vi "main.vi"() -> ()   [LabVIEW 2013]
doc: "Use this template to build a producer/consumer design pattern with events to produce queue items. Use this design pattern instead of the User Interface Event Handler pattern for user interfaces when you want to execute code asynchronously in response to an event without slowing the user interface responsiveness."
uses:
  Microscope_Settings.ctl
  Laser.ctl
  Time_microseconds.ctl
  Phase_Shift.ctl
  Mirror_Voltage.ctl
  Z_Offset.ctl
  Gain.ctl
  Tuneable_Lens_Numeric_Control.ctl
  Piezo_micrometres.ctl
  waveforms.ctl
  Piezo_micrometres_slider_control.ctl
  Mirror_Gain_Slider_Control.ctl
  Tunable_Lens_Slider_Control.ctl
panel:
  in  "COM port":i32
  in  "Filter Wheel Position":i32
  in  "Mode":T1(ring)
  in  "Number of Repetitions":u16=1 min=1 step=1
  in  "Time Interval  Between Repeats (µS)":T2 step=2
  in  "StopMultiDScan":bool
  in  "StartMultiDScan":bool
  in  "Number of Z Slices":i16=1 min=1 step=1
  in  "Z Mirror Control":enum16{"manual", "automatic"}(ring)
  in  "Apply ex/det correction":enum16{"no", "yes"}(ring)
  out "Z Mirror Voltage":T3 min=-10.0 max=10.0
  out "Adjusted Scan Mirror Voltage":T3 min=-10.0 max=10.0
  in  "set@minZ":bool
  in  "set@maxZ":bool
  in  "@ min Z":T3 min=-10.0 max=10.0
  in  "@ max Z":T3 min=-10.0 max=10.0
  in  "PiezoEndMicrometres":T4 caption="End (µm)" min=0.0 max=100.0
  in  "PiezoStartMicrometres":T4 caption="Start (µm)" min=0.0 max=100.0
  in  "setPiezoEnd":bool
  in  "setPiezoStart":bool
  in  "Lens 2":T5 min=0.0 max=3.0 step=0.0001 scale=0.0..3.0
  in  "Lens 1":T5 min=0.0 max=3.0 step=0.0001 scale=0.0..3.0
  in  "saveMicroscopeSettings":bool
  in  "applyCurrentMicroscopeSettings":bool
  in  "deleteCurrentMicroscopeSettings":bool
  in  "loadMicroscopeSettings":bool
  in  "addMicroscopeSettings":bool
  in  "Z Mirror Gain":T6 min=-10.0 max=10.0 scale=-10.0..10.0
  in  "Mirror Offset":dbl(slide) min=-10.0 max=10.0 step=0.01 scale=-10.0..10.0
  in  "Laser":T7
  in  "Piezo Position (µm)":T8 min=0.0 max=100.0 scale=0.0..100.0
  in  "Mirror Voltage":dbl(slide) min=-10.0 max=10.0 step=0.01 scale=-10.0..10.0
  in  "setPosition2":bool
  in  "setPosition1":bool
  in  "Z offset 2":T9
  in  "Z offset 1":T9
  in  "Scan Mirror 2":T3 min=-10.0 max=10.0
  in  "Scan Mirror 1":T3 min=-10.0 max=10.0
  in  "setScanMirrorMin":bool
  in  "setScanMirrorMax":bool
  in  "MinScanMirror":T3 caption="Min" min=-10.0 max=10.0
  in  "MaxScanMirror":T3 caption="Max" min=-10.0 max=10.0
  in  "Offset":T3 min=-10.0 max=10.0
  in  "Amplitude":T3 min=-10.0 max=10.0
  in  "Phase Shift (µS)":i32(slide) scale=-5000.0..1000.0
  in  "Sweep Interval (µS)":T2 step=2
  in  "Sweep Time (µS)":T2 step=20
  in  "Microscope Settings":T10[](array[typedef]) {"Number Z Slices" min=1 step=1; "Piezo End (µm)" min=0.0 max=100.0; "Piezo Start (µm)" min=0.0 max=100.0; "Beam @ max Z" min=-10.0 max=10.0; "Beam @ min Z" min=-10.0 max=10.0; "Tuneable Lens 2" min=0.0 max=3.0 step=0.0001; "Tuneable Lens 1" min=0.0 max=3.0 step=0.0001; "Scan Mirror Position 2" min=-10.0 max=10.0; "Scan Mirror Position 1" min=-10.0 max=10.0; "Scan Mirror Amplitude" min=-10.0 max=10.0; "Scan Mirror Min" min=-10.0 max=10.0; "Scan Mirror Max" min=-10.0 max=10.0; "Sweep Interval (µS)" step=2; "Sweep Time (µS)" step=2}
  in  "Sample Rate (kHz)":i32
  in  "StopSinglePlaneScan":bool
  in  "StartSinglePlaneScan":bool
  in  "exit":bool
  # "Piezo Settings"
  # "Scan Mirror Settings"
  # "Z Mirror Local Settings"
  # "Single Plane Scan"
  # "Multidimensional Scan"
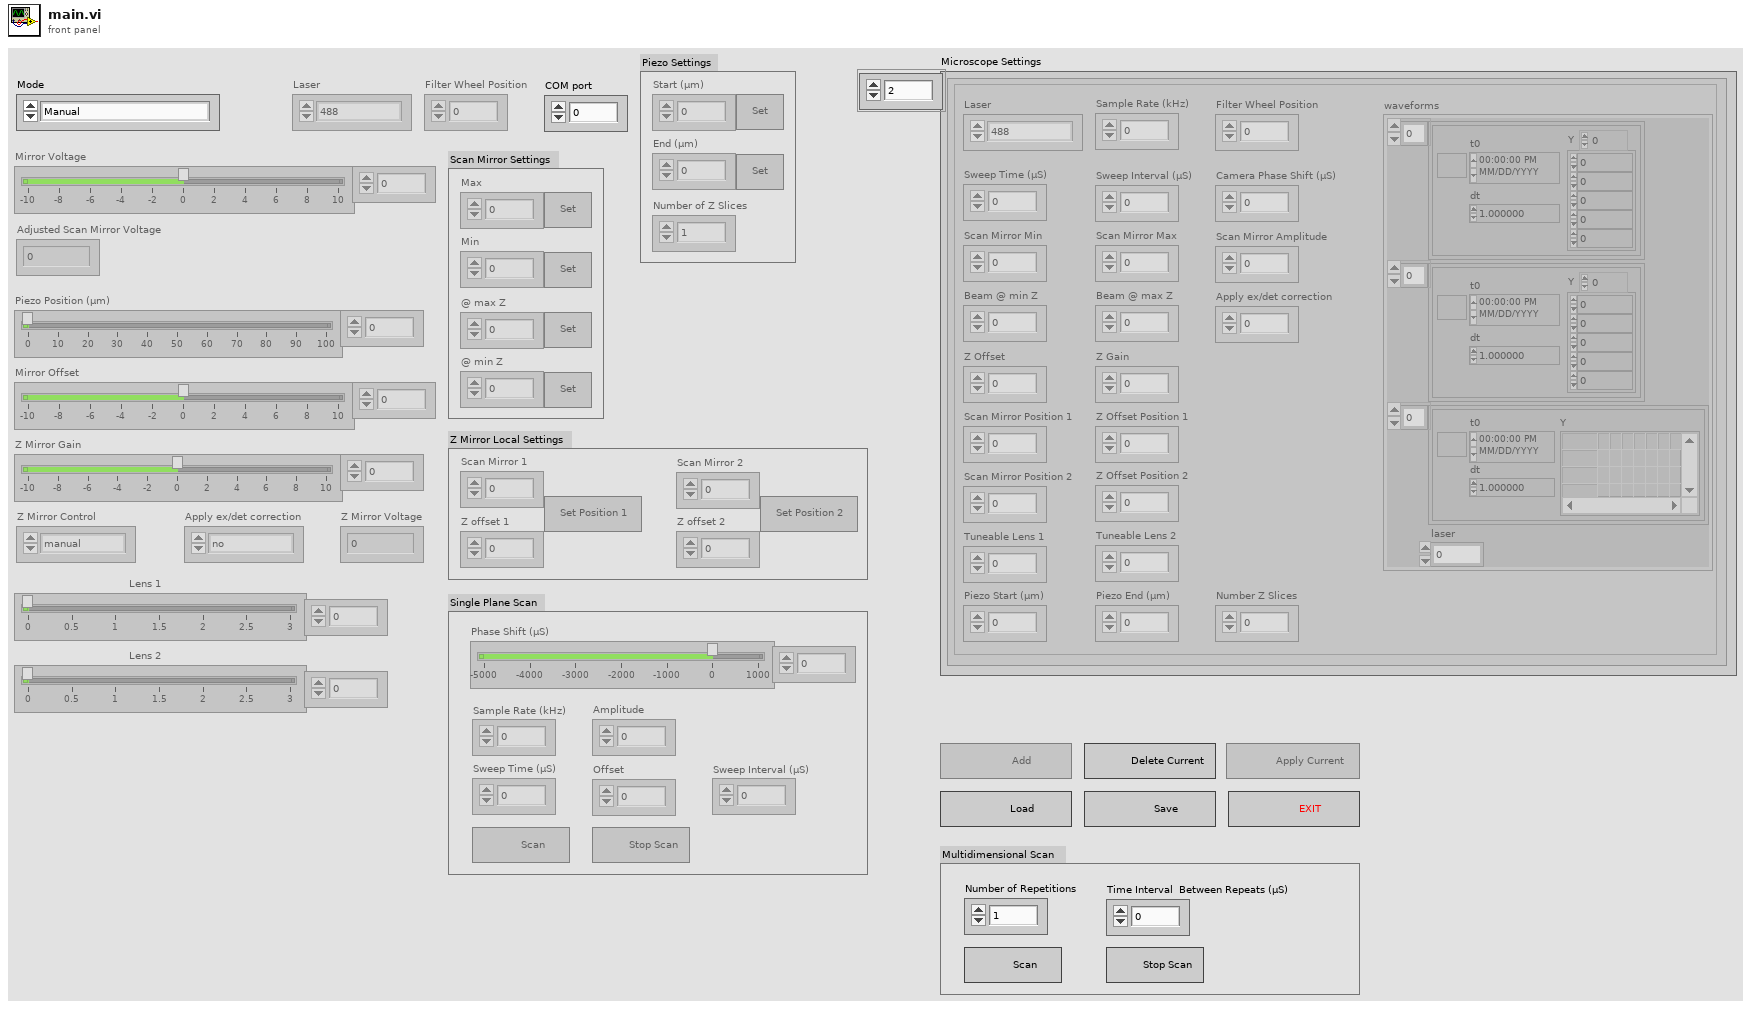
[diagram p1: front panel]
types:
  T1 = enum8{"Manual", "Single Plane Scan", "Multi-Dimensional Scan"}
  T2 = typedef "Time_microseconds.ctl" = u32
  T3 = typedef "Mirror_Voltage.ctl" = dbl
  T4 = typedef "Piezo_micrometres.ctl" = dbl
  T5 = typedef "Tunable_Lens_Slider_Control.ctl" = dbl
  T6 = typedef "Mirror_Gain_Slider_Control.ctl" = dbl
  T7 = typedef "Laser.ctl" = enum16{"488", "561"}
  T8 = typedef "Piezo_micrometres_slider_control.ctl" = dbl
  T9 = typedef "Z_Offset.ctl" = dbl
  T10 = typedef "Microscope_Settings.ctl" = cluster{"Laser":T7, "Sweep Time (µS)":T2, "Sweep Interval (µS)":T2, "Sample Rate (kHz)":dbl, "Camera Phase Shift (µS)":T11, "Scan Mirror Max":T3, "Scan Mirror Min":T3, "Scan Mirror Amplitude":T3, "Z Offset":T9, "Z Gain":T12, "Scan Mirror Position 1":T3, "Z Offset Position 1":T9, "Scan Mirror Position 2":T3, "Z Offset Position 2":T9, "Tuneable Lens 1":T13, "Tuneable Lens 2":T13, "Beam @ min Z":T3, "Beam @ max Z":T3, "Piezo Start (µm)":T4, "Piezo End (µm)":T4, "Number Z Slices":i16, "Filter Wheel Position":i32, "Apply ex/det correction":u16, "waveforms":T14}
  T11 = typedef "Phase_Shift.ctl" = i32
  T12 = typedef "Gain.ctl" = dbl
  T13 = typedef "Tuneable_Lens_Numeric_Control.ctl" = dbl
  T14 = typedef "waveforms.ctl" = cluster{waveform(dbl)[], waveform(dbl)[], digitalwaveform[], "laser":i32}
  T15 = enum8{"Enabled", "Disabled", "Disabled and Grayed Out"}
  T16 = enum16{"deny read/write", "deny write-only", "deny none"}
  T17 = enum16{"open", "replace", "create", "open or create", "replace or create", "replace or create with confirmation"}
  T18 = cluster{"Laser":T7, "Sweep Time (µS)":T2, "Sweep Interval (µS)":T2, "Sample Rate (kHz)":i32, "Phase Shift (µS)":i32, "MaxScanMirror":T3, "MinScanMirror":T3, "MaxScanMirror":T3, "Mirror Offset":dbl, "Z Mirror Gain":T6, "Scan Mirror 1":T3, "Z offset 1":T9, "Scan Mirror 2":T3, "Z offset 2":T9, "Lens 1":T5, "Lens 2":T5, "@ min Z":T3, "@ max Z":T3, "PiezoStartMicrometres":T4, "PiezoEndMicrometres":T4, "Number of Z Slices":i16, "Filter Wheel Position":i32, "Apply ex/det correction":enum16{"no", "yes"}}
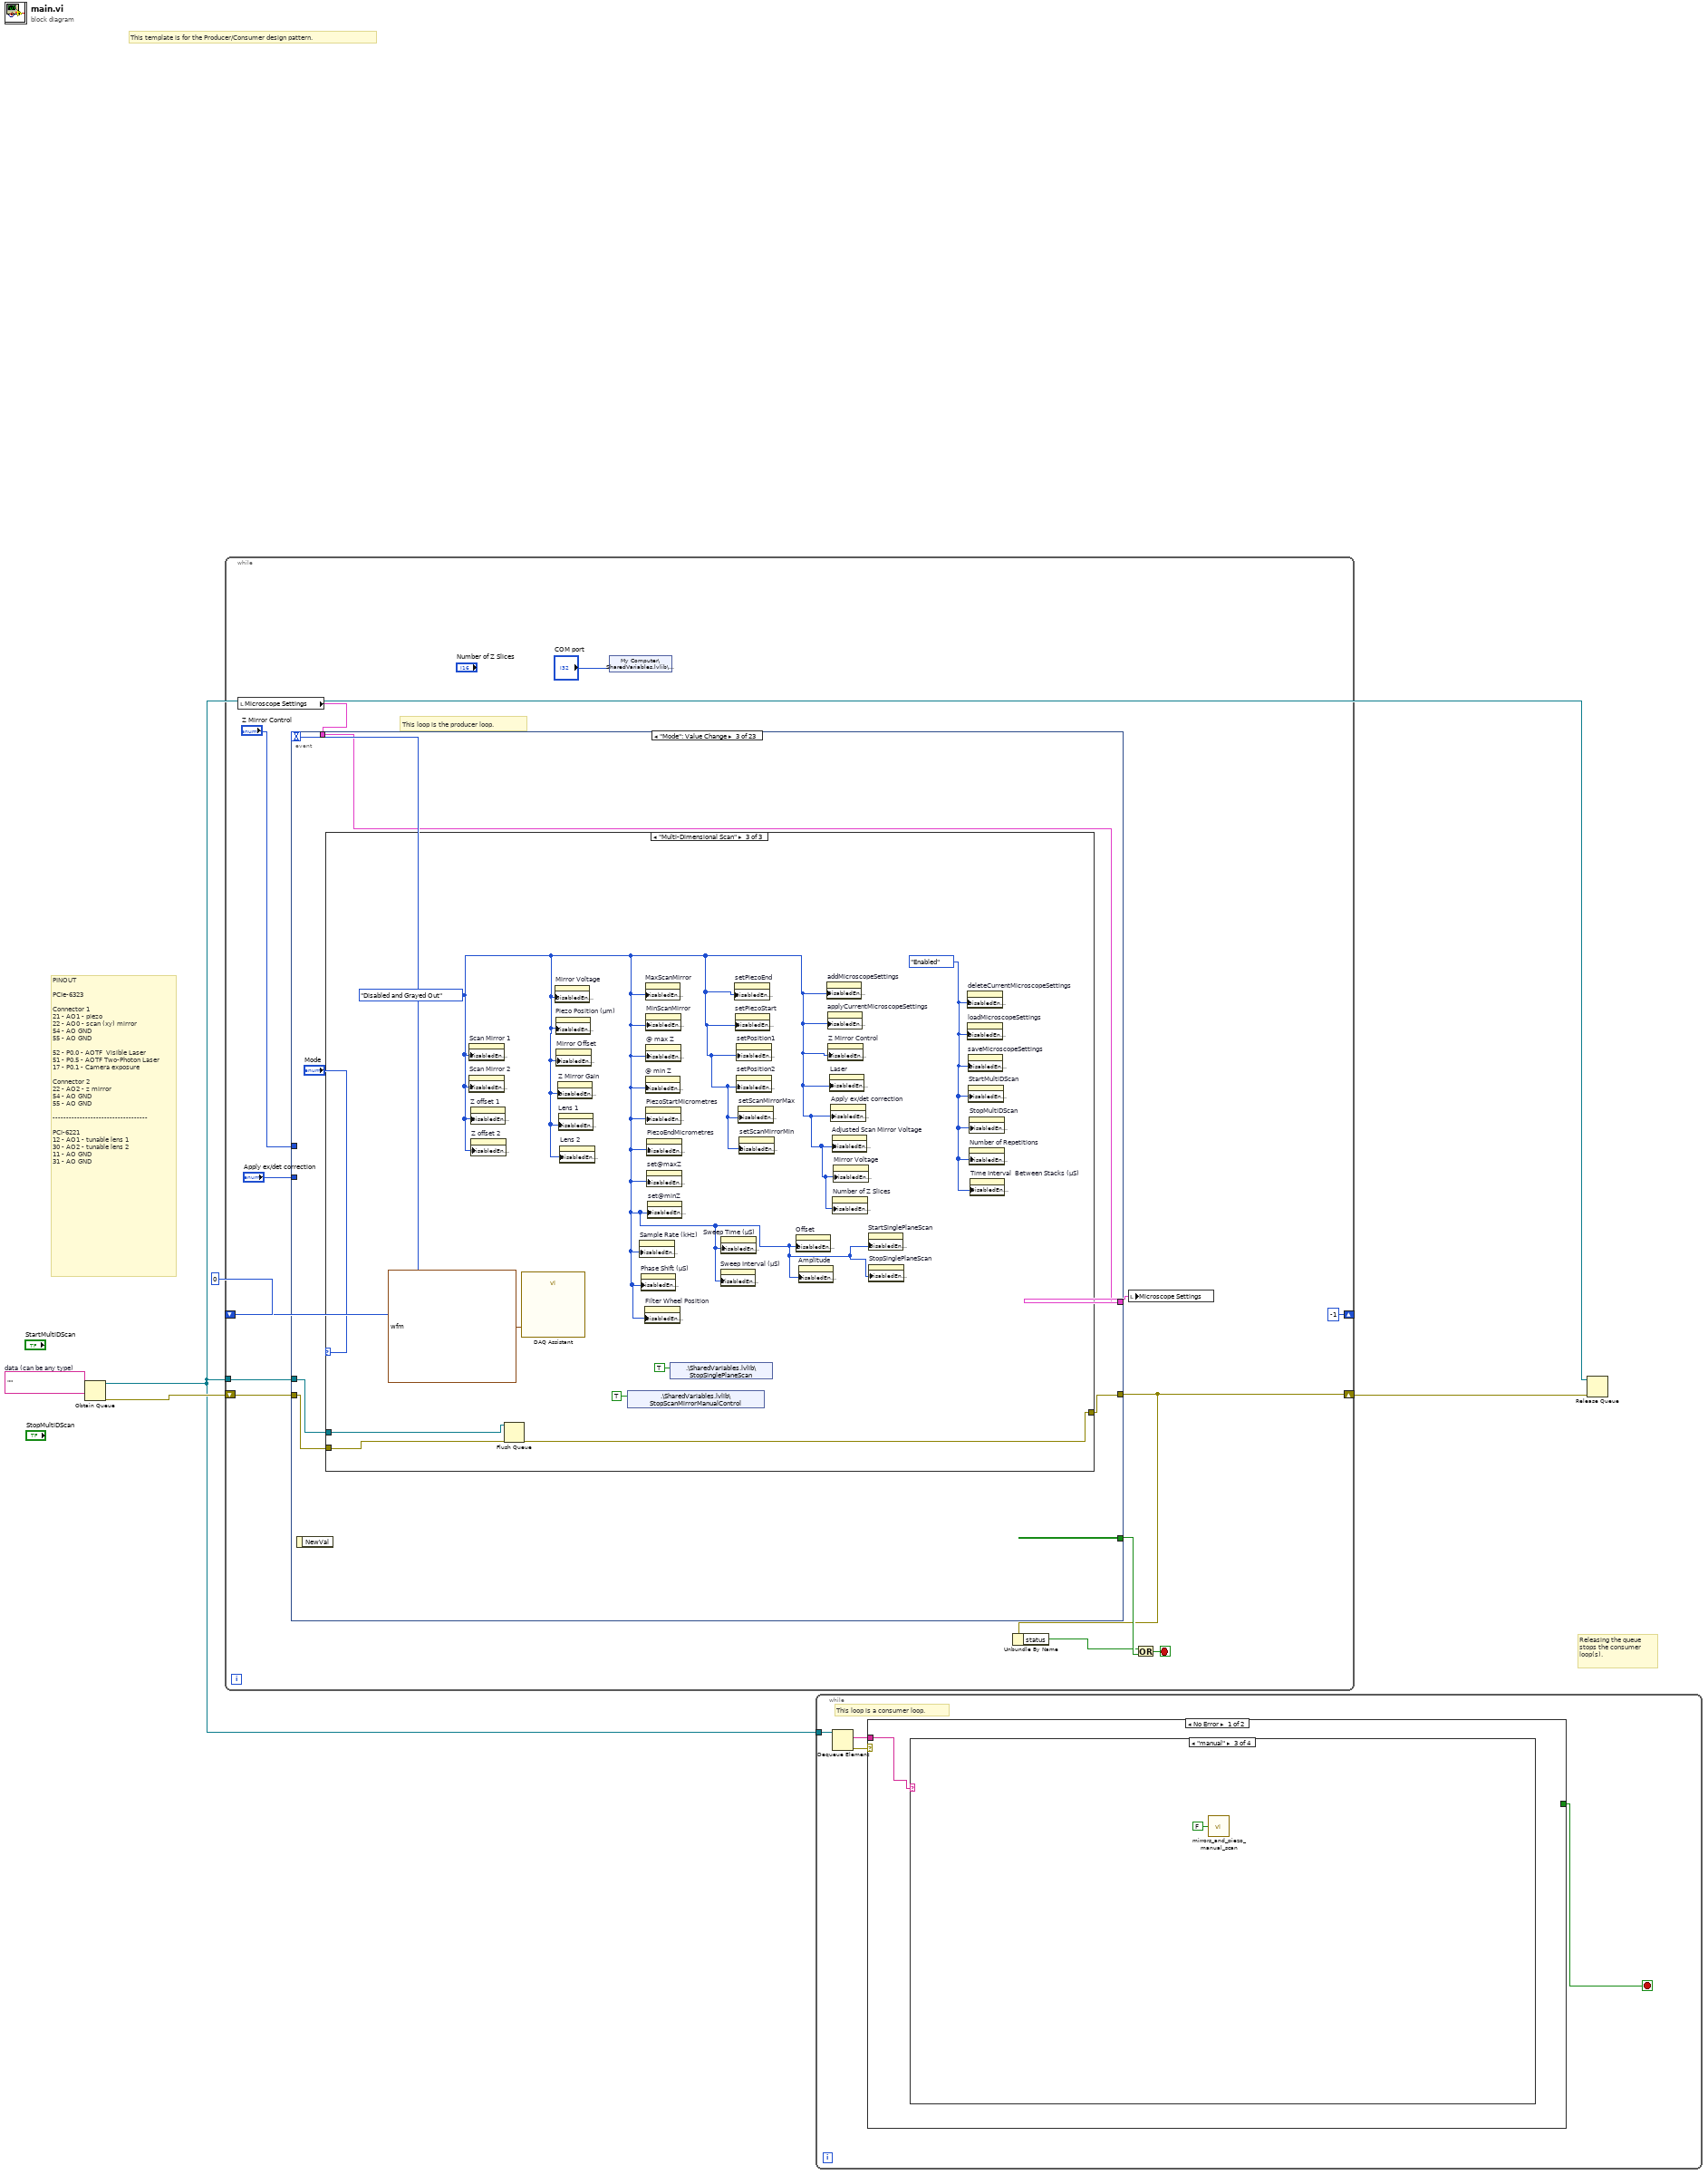
[diagram p0: block diagram]
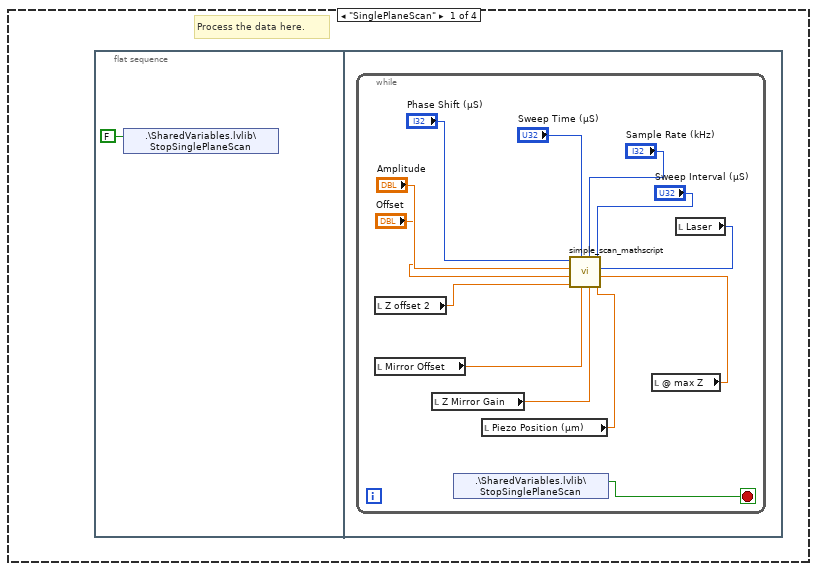
[diagram p2: hidden frame]
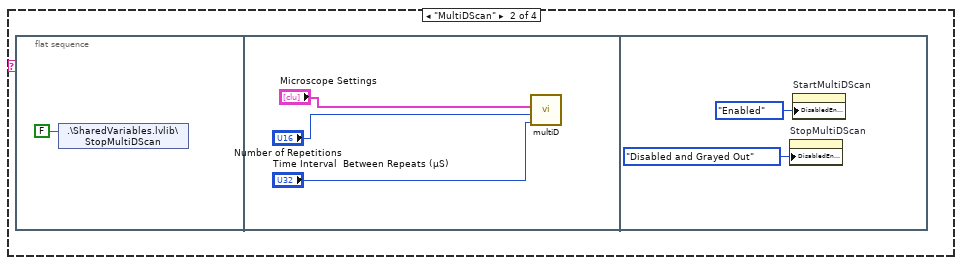
[diagram p3: hidden frame]
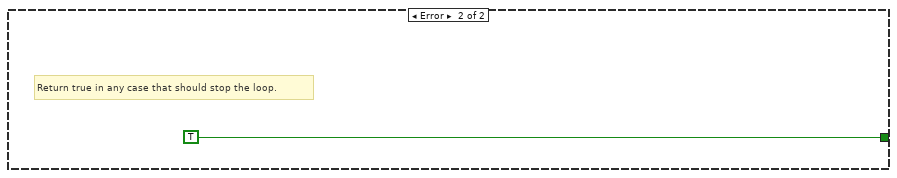
[diagram p5: hidden frame]
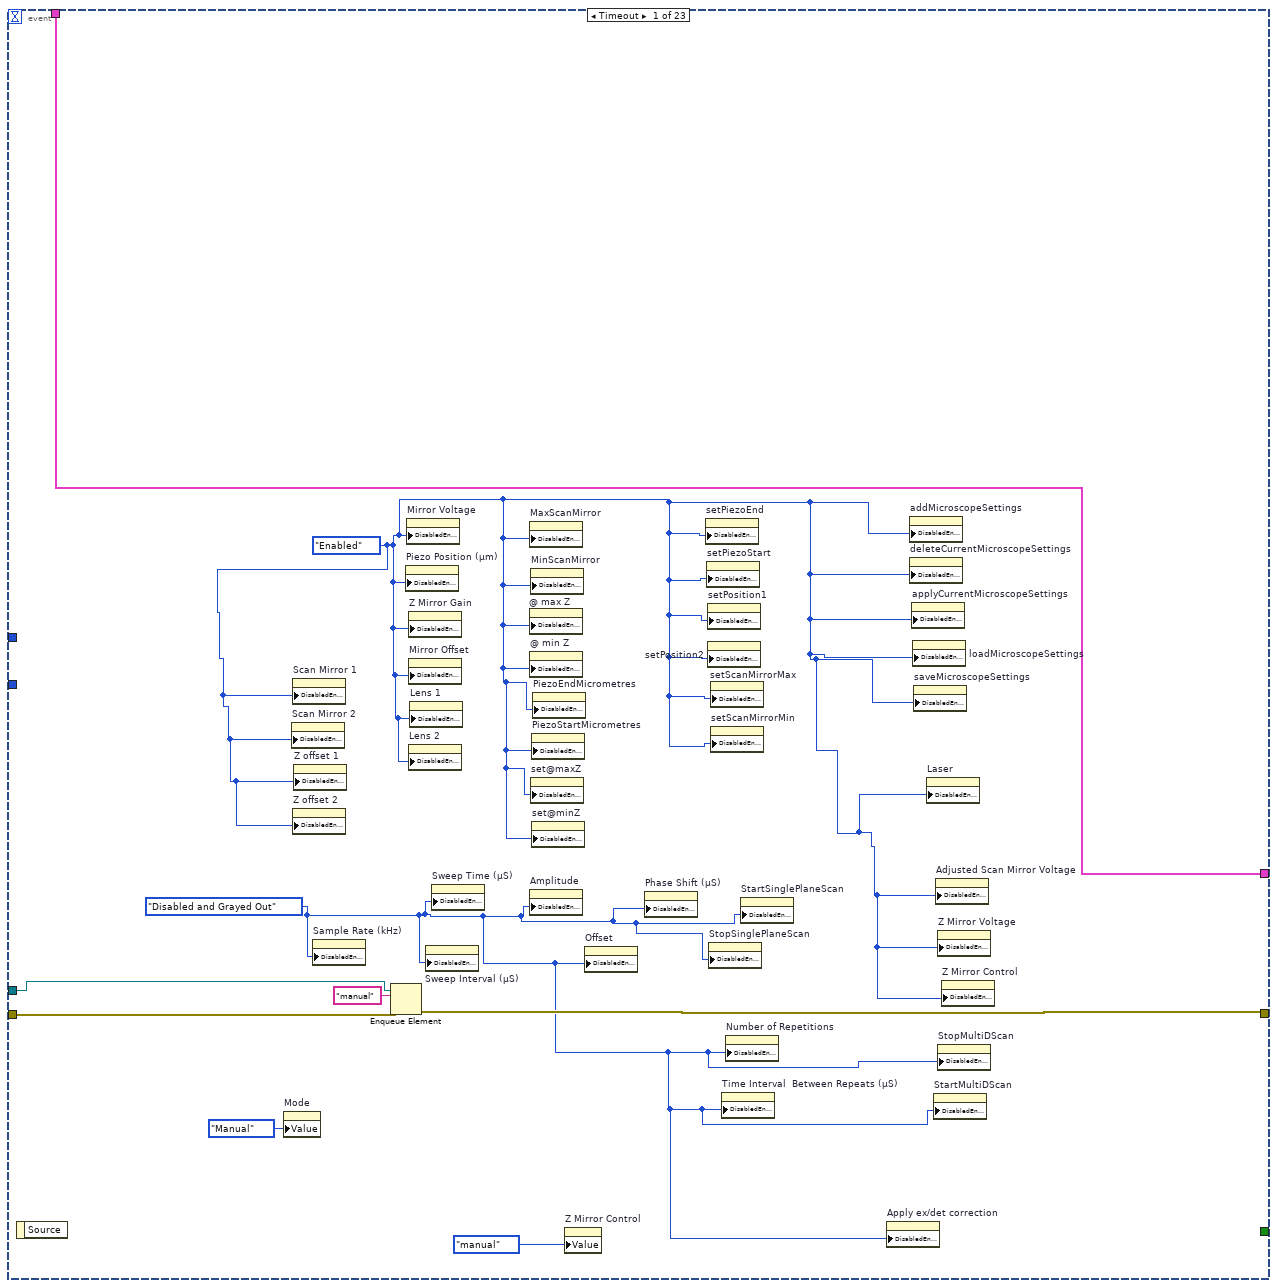
[diagram p6: hidden frame]
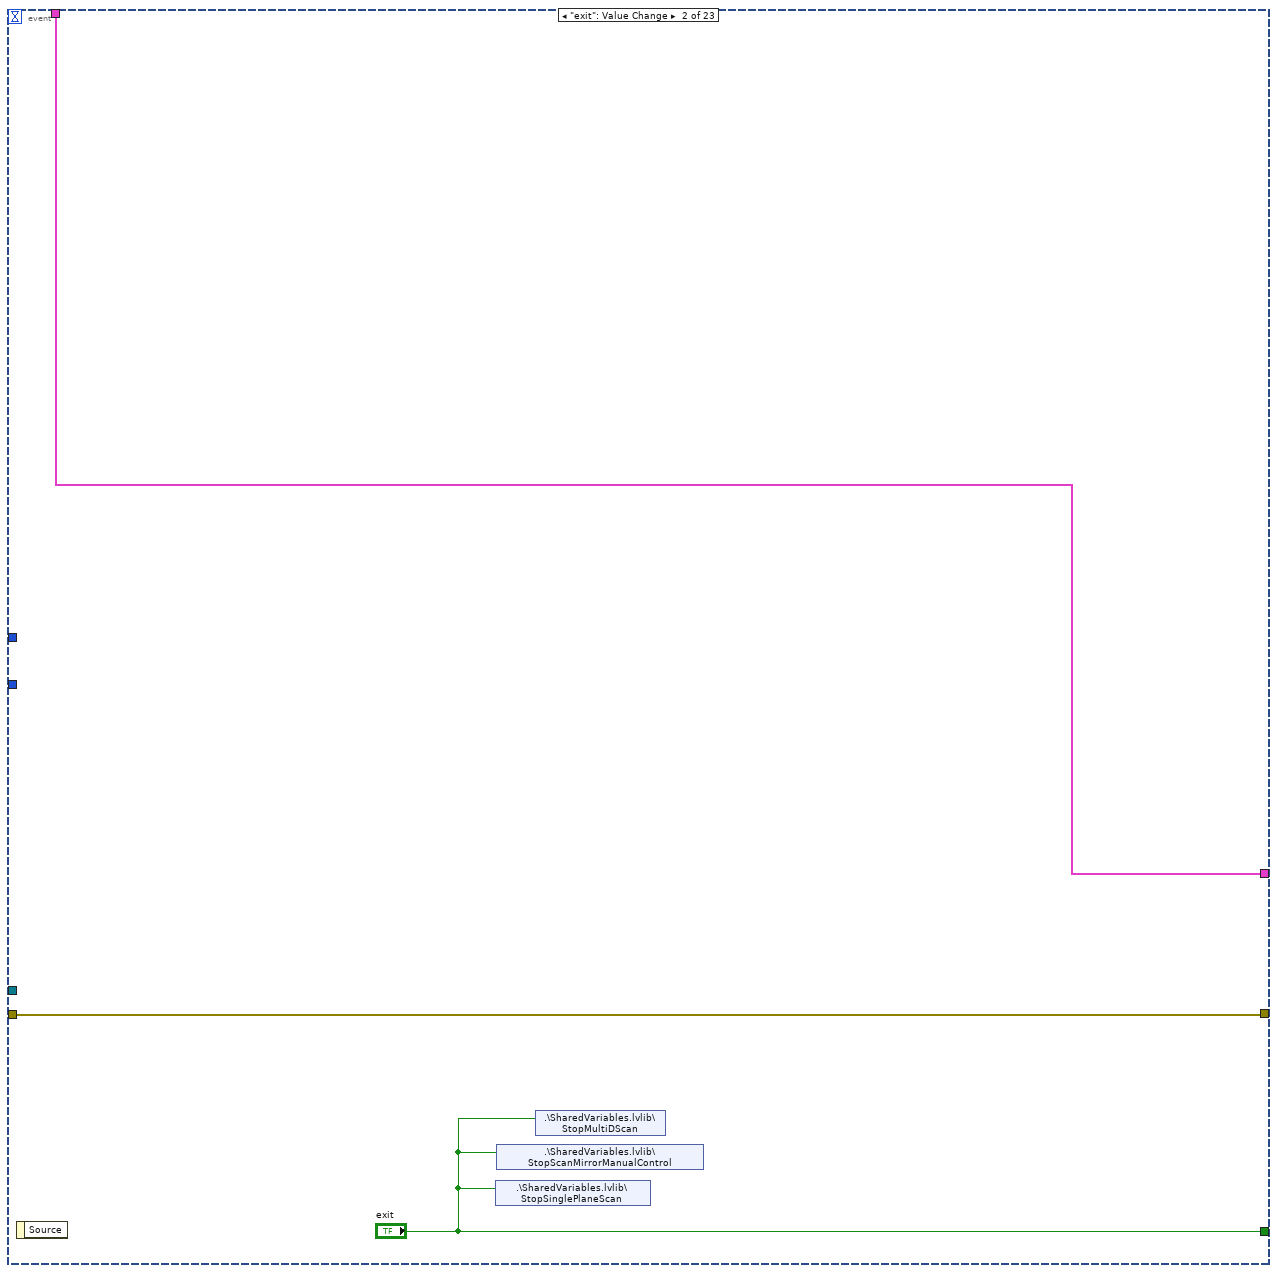
[diagram p7: hidden frame]
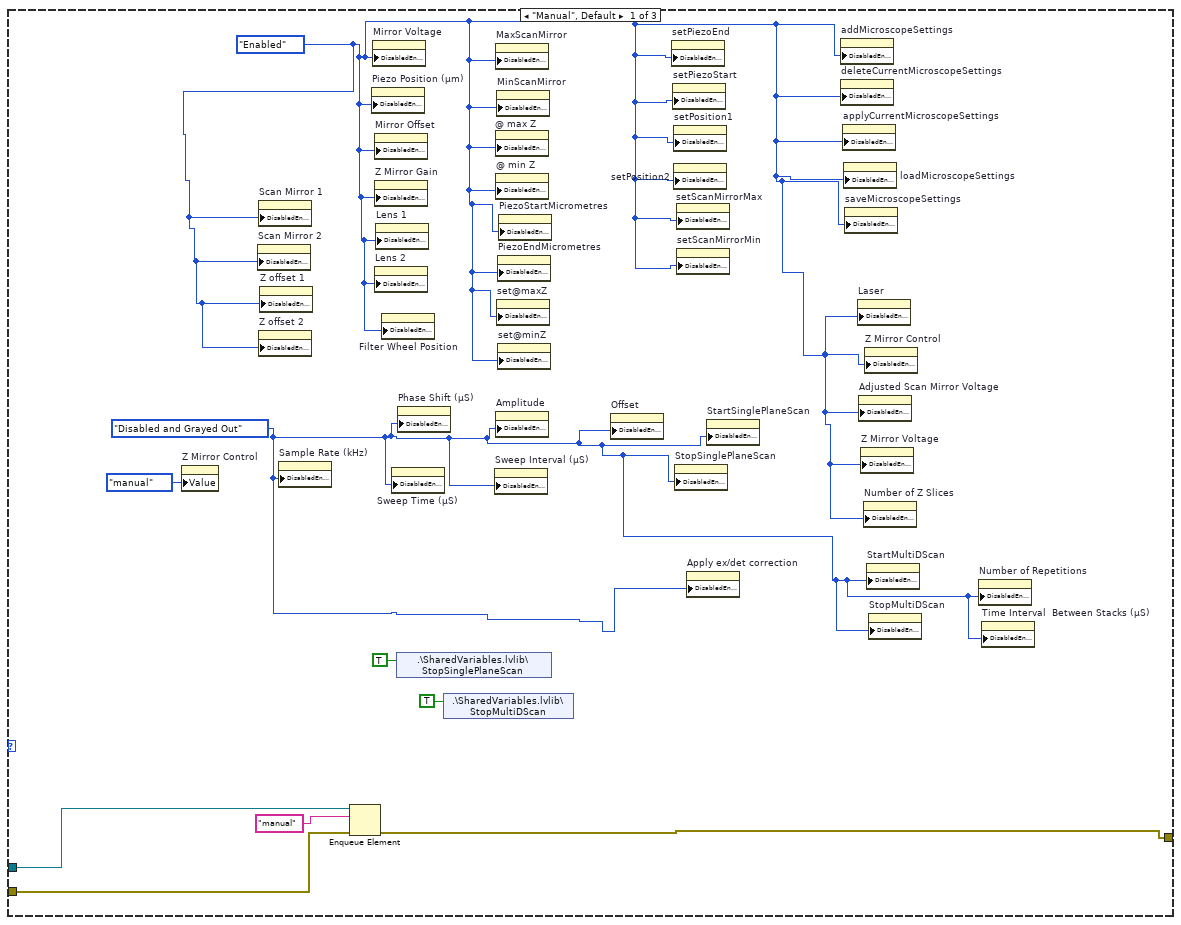
[diagram p8: hidden frame]
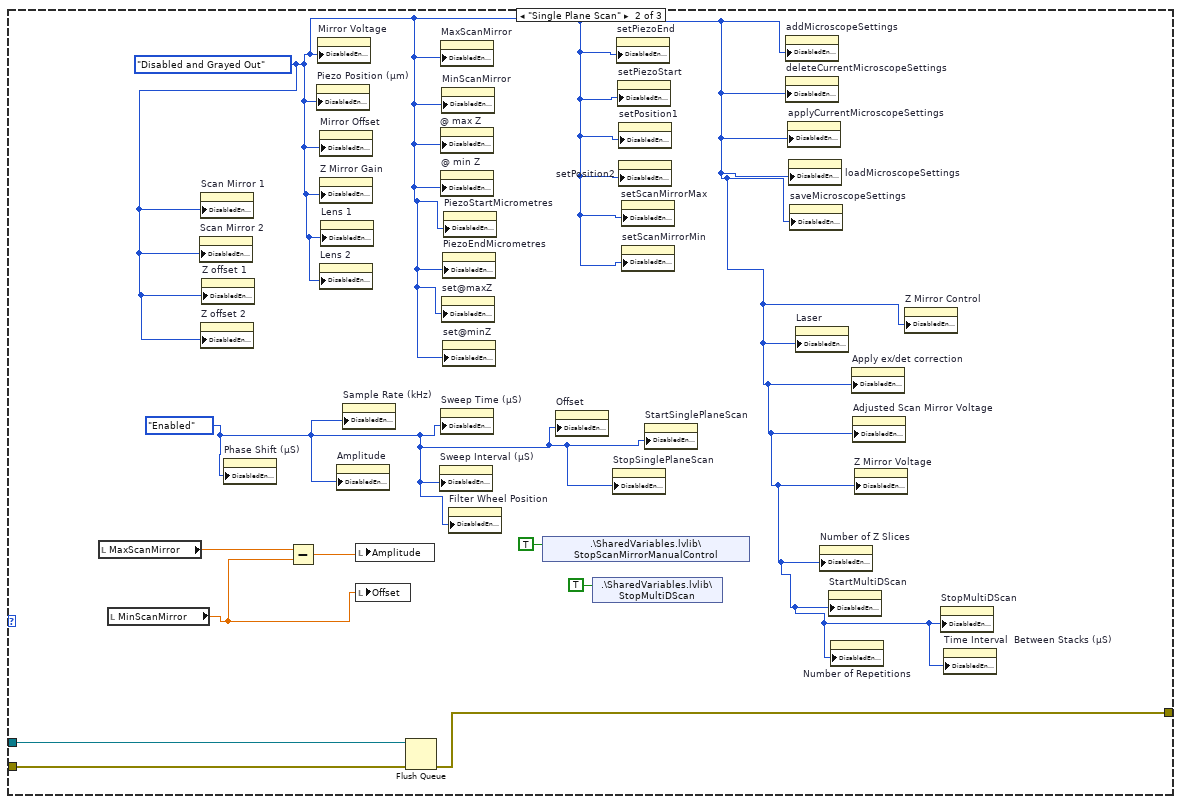
[diagram p9: hidden frame]
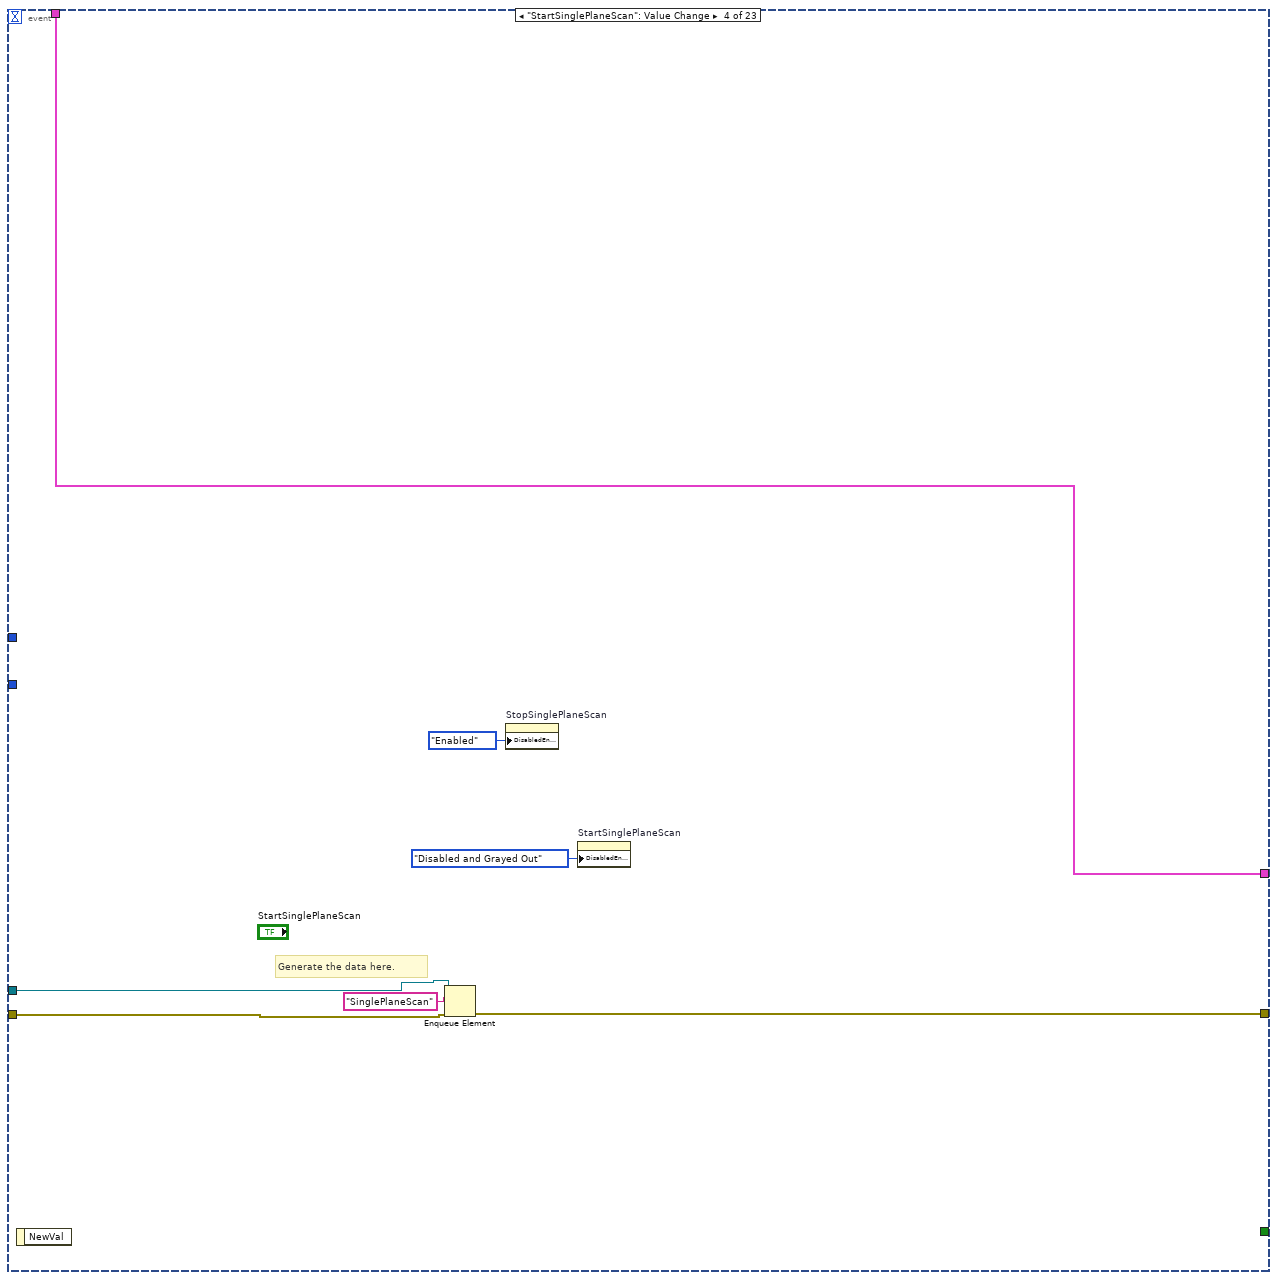
[diagram p10: hidden frame]
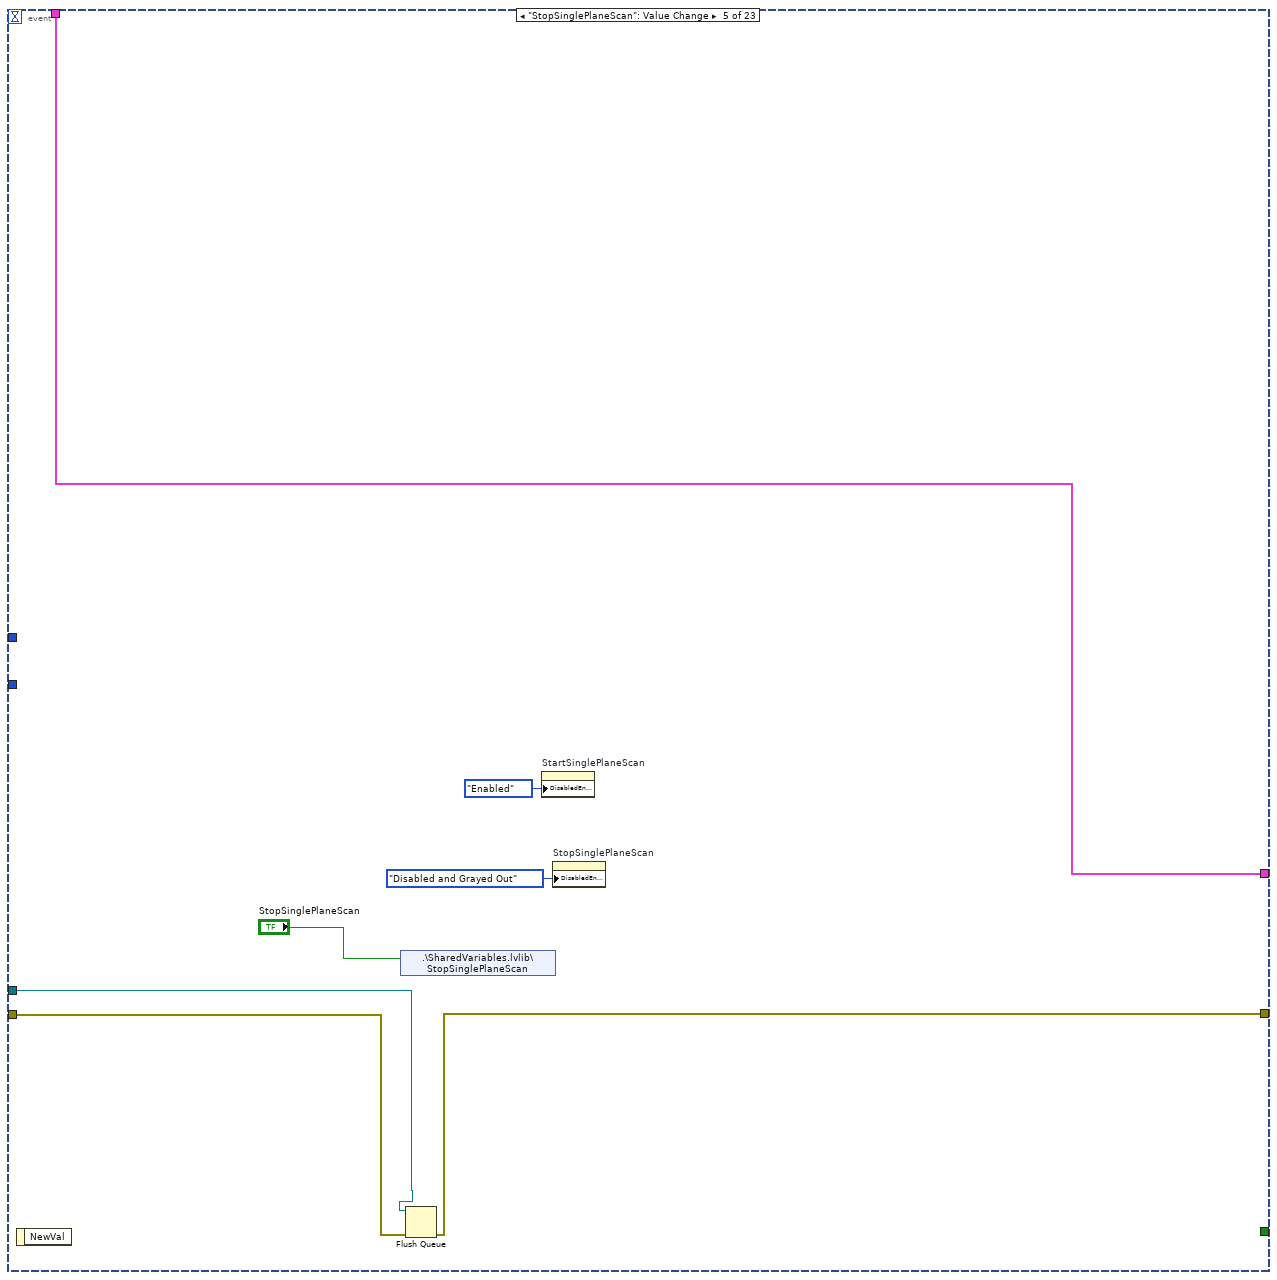
[diagram p11: hidden frame]
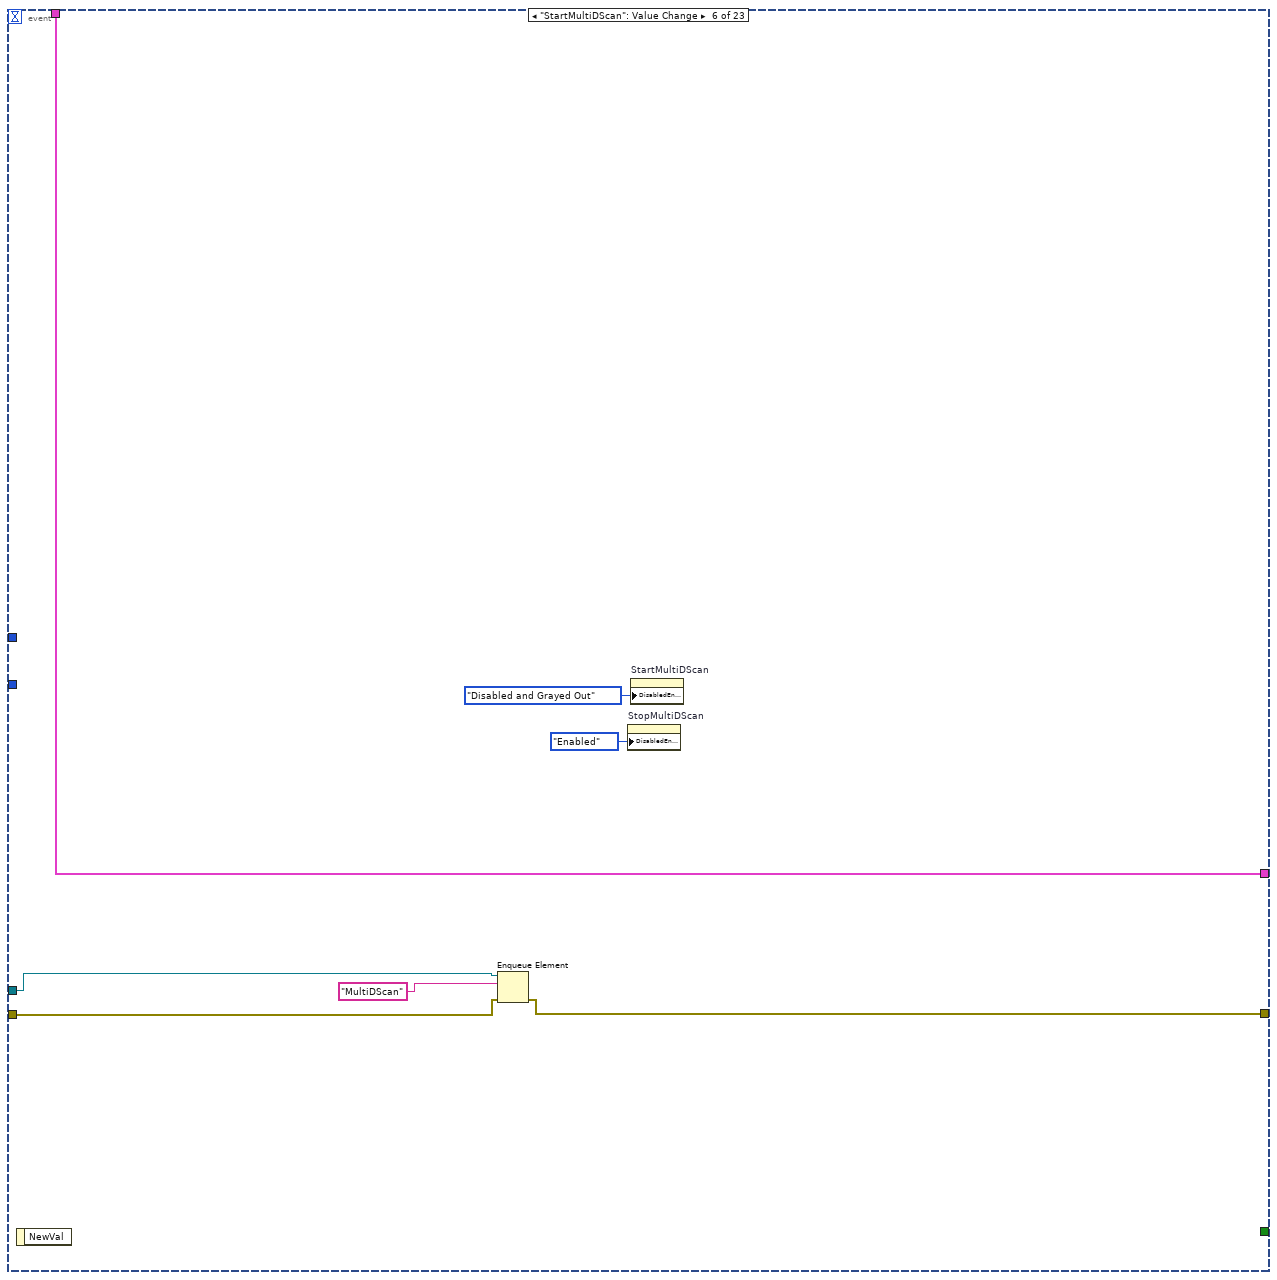
[diagram p12: hidden frame]
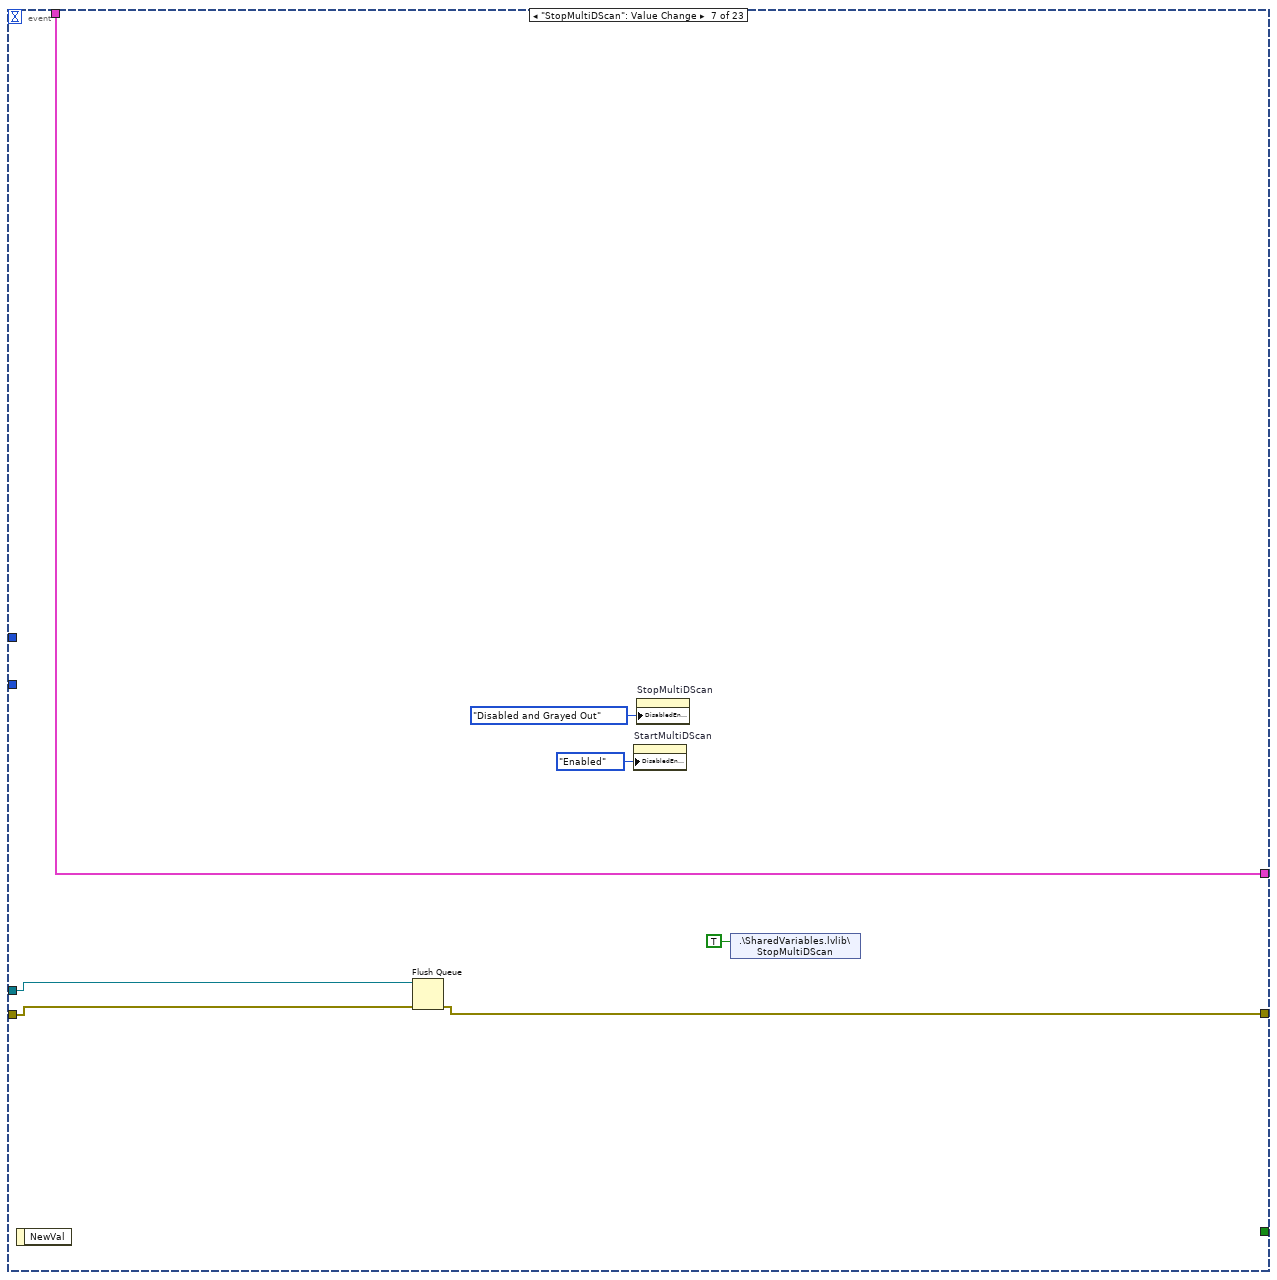
[diagram p13: hidden frame]
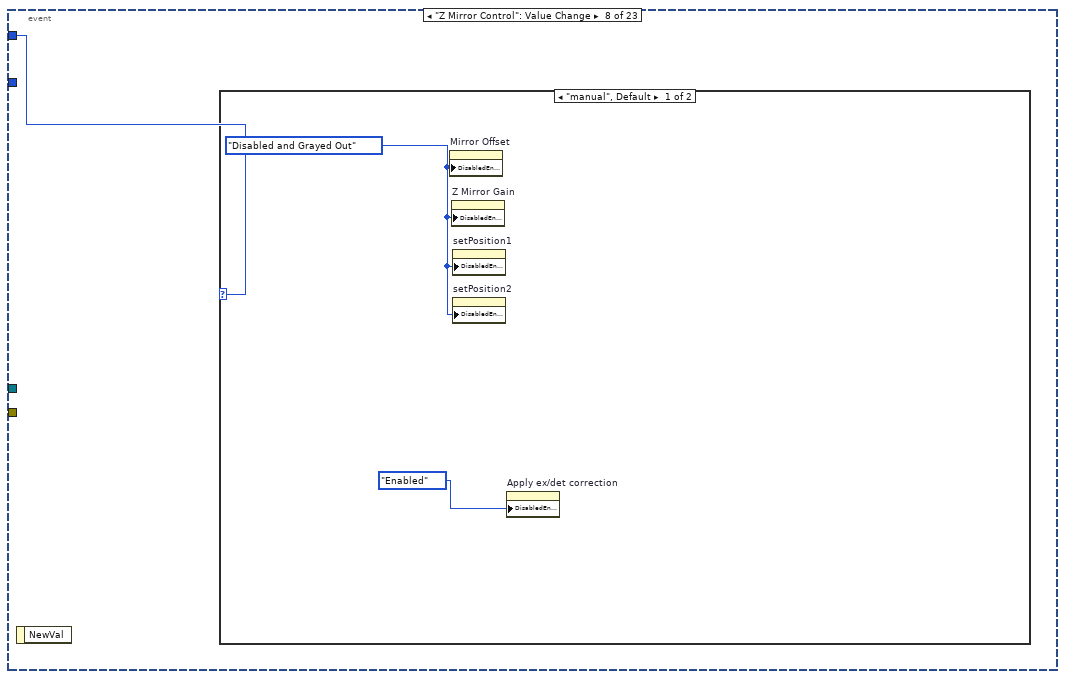
[diagram p14: hidden frame]
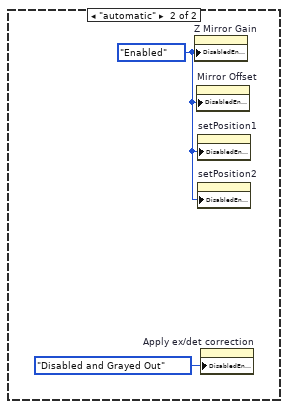
[diagram p15: hidden frame]
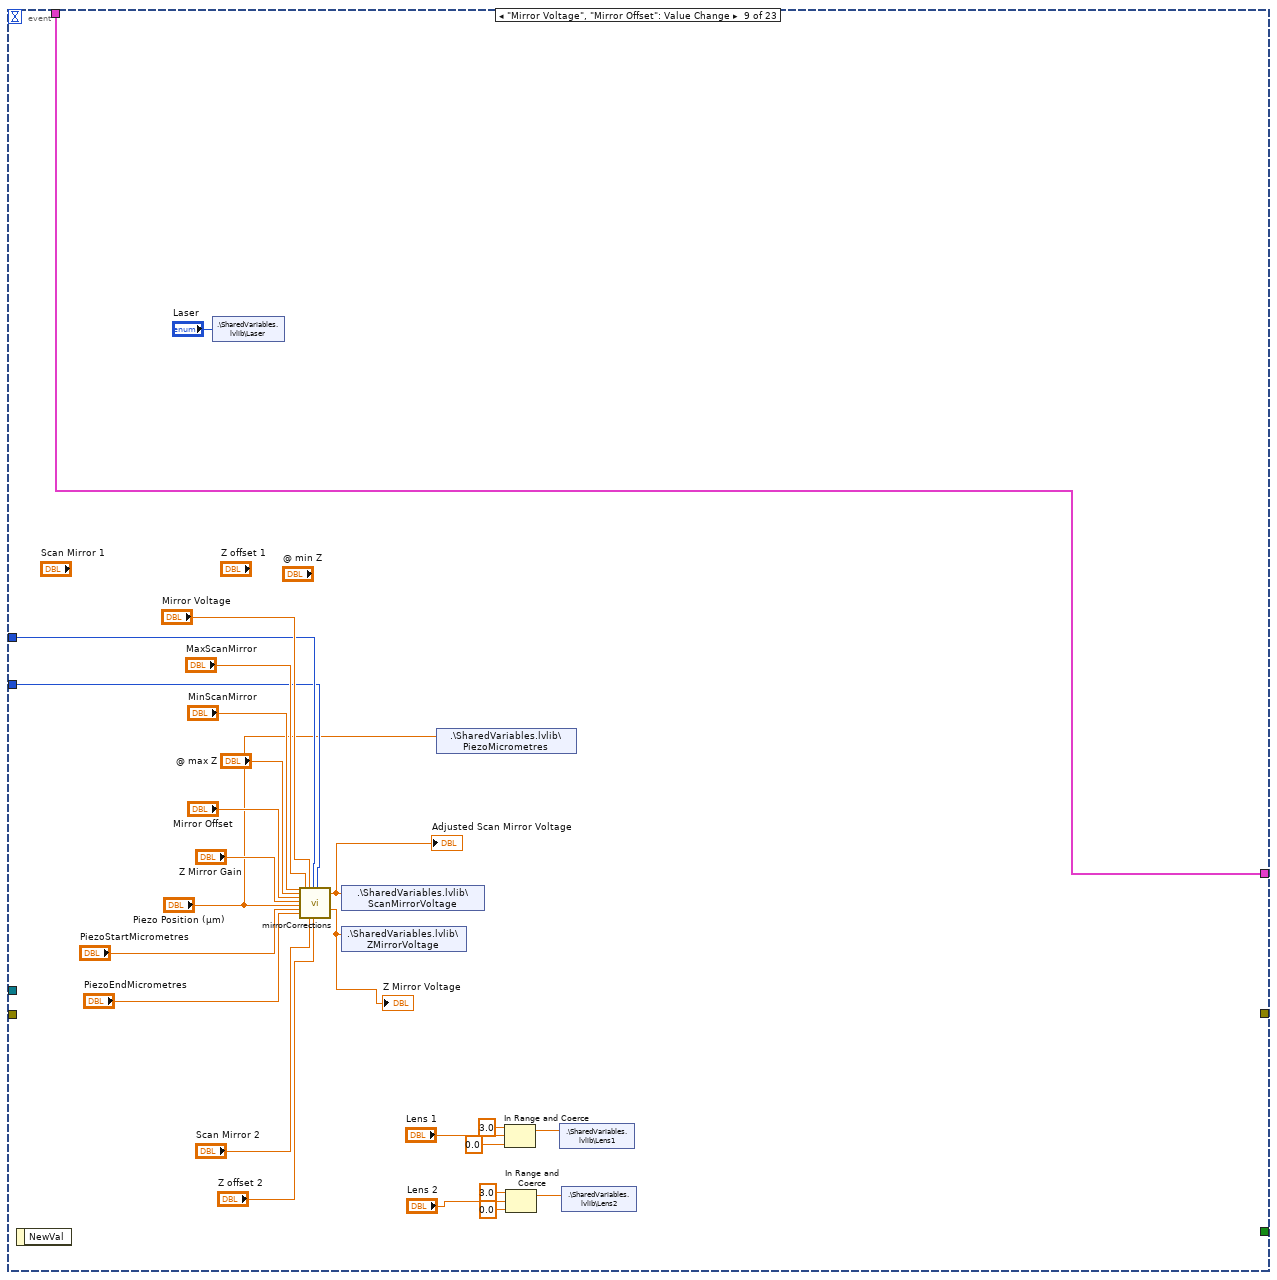
[diagram p16: hidden frame]
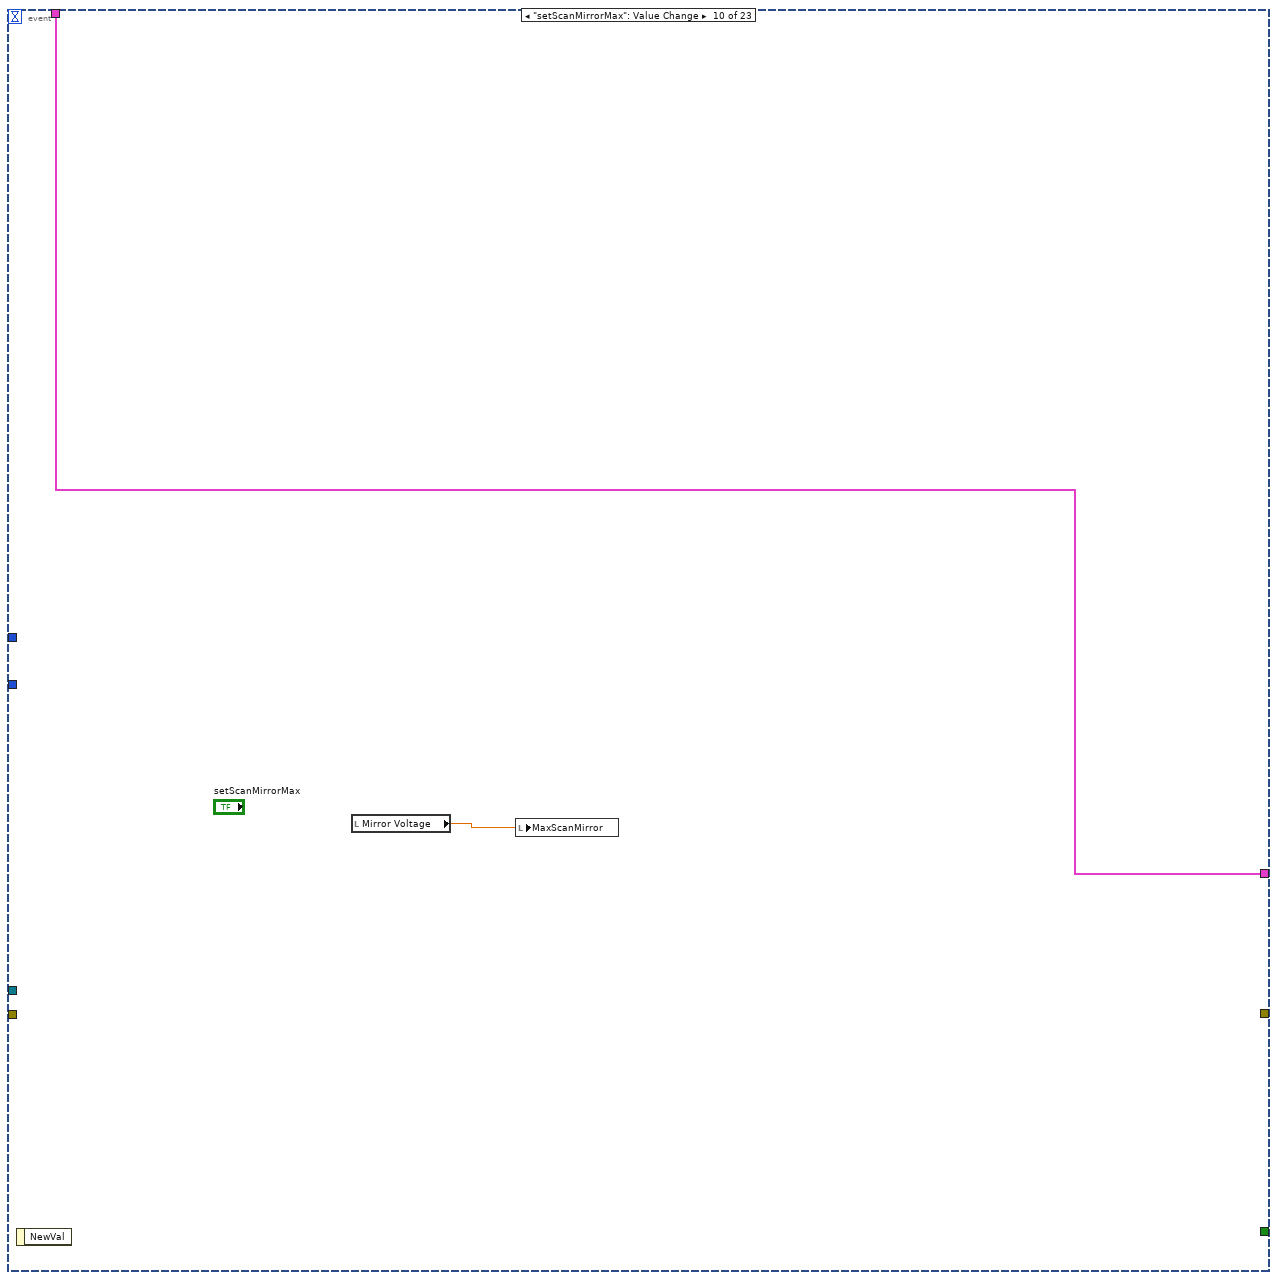
[diagram p17: hidden frame]
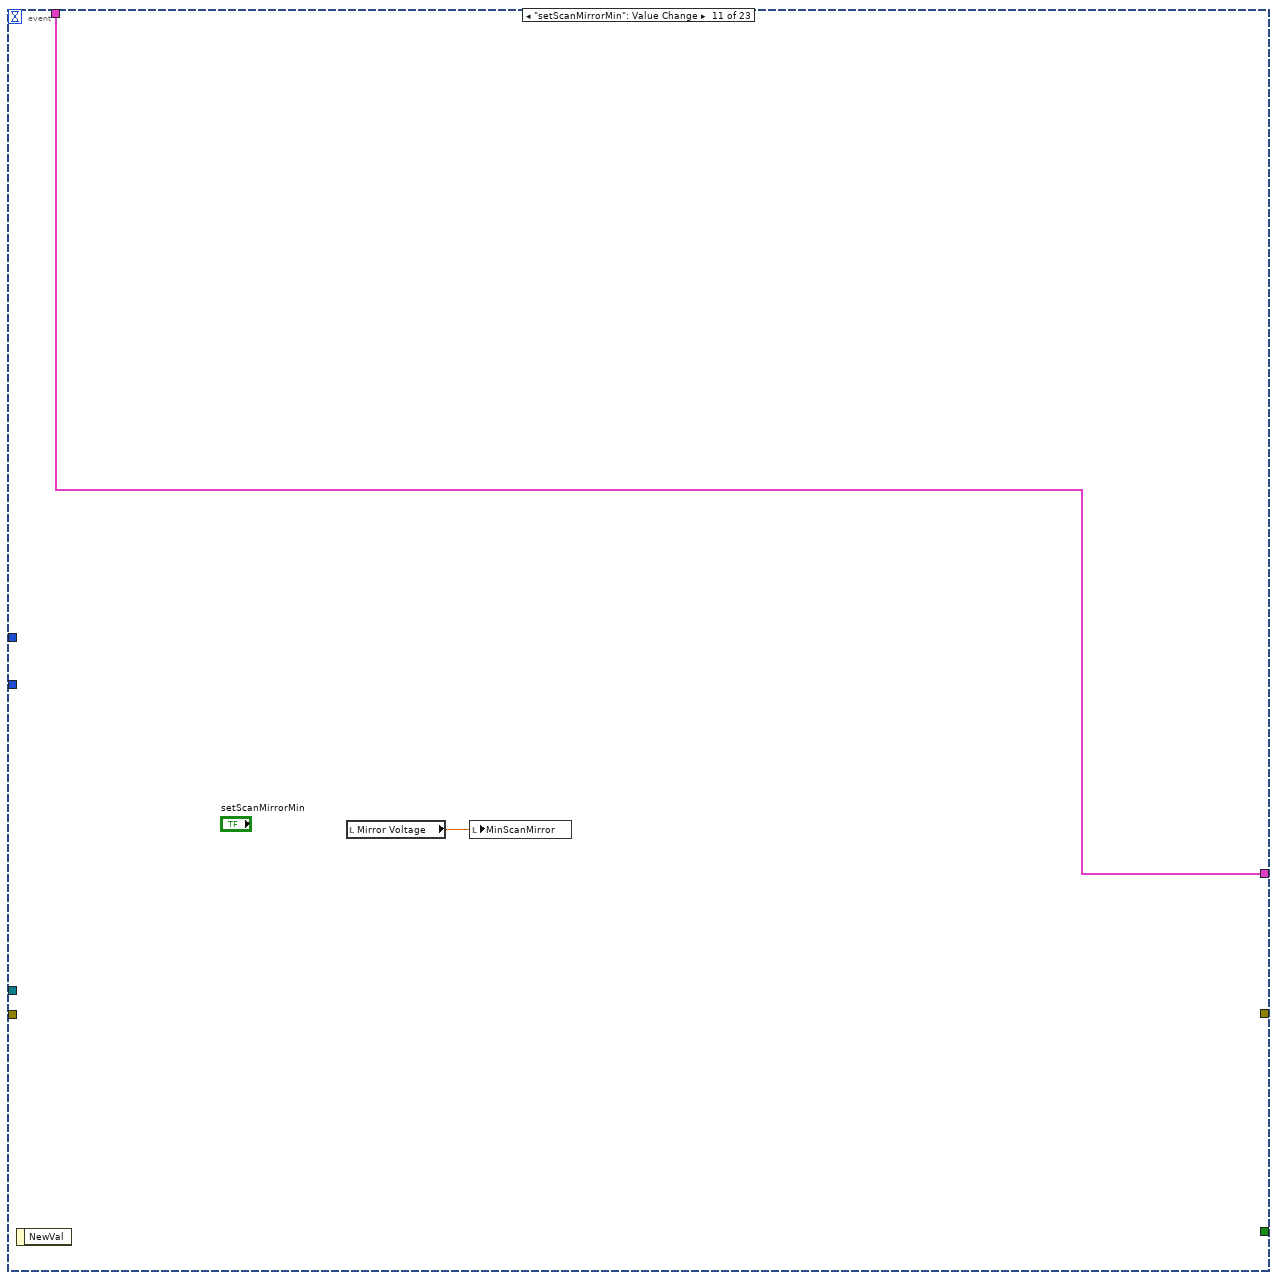
[diagram p18: hidden frame]
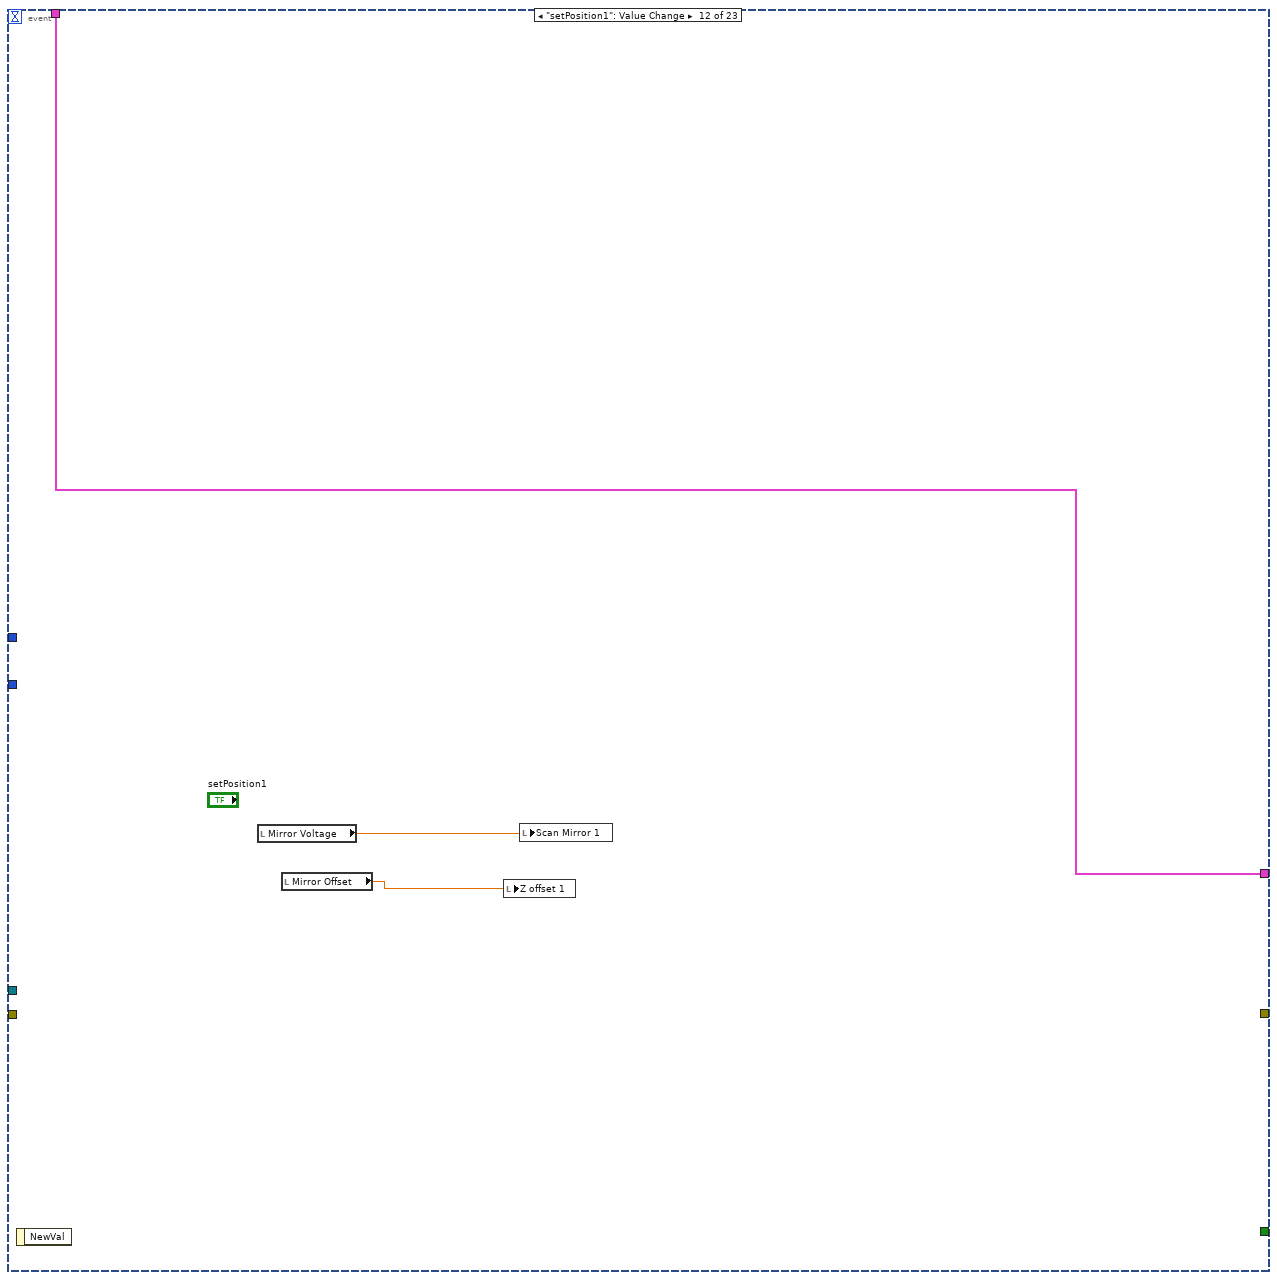
[diagram p19: hidden frame]
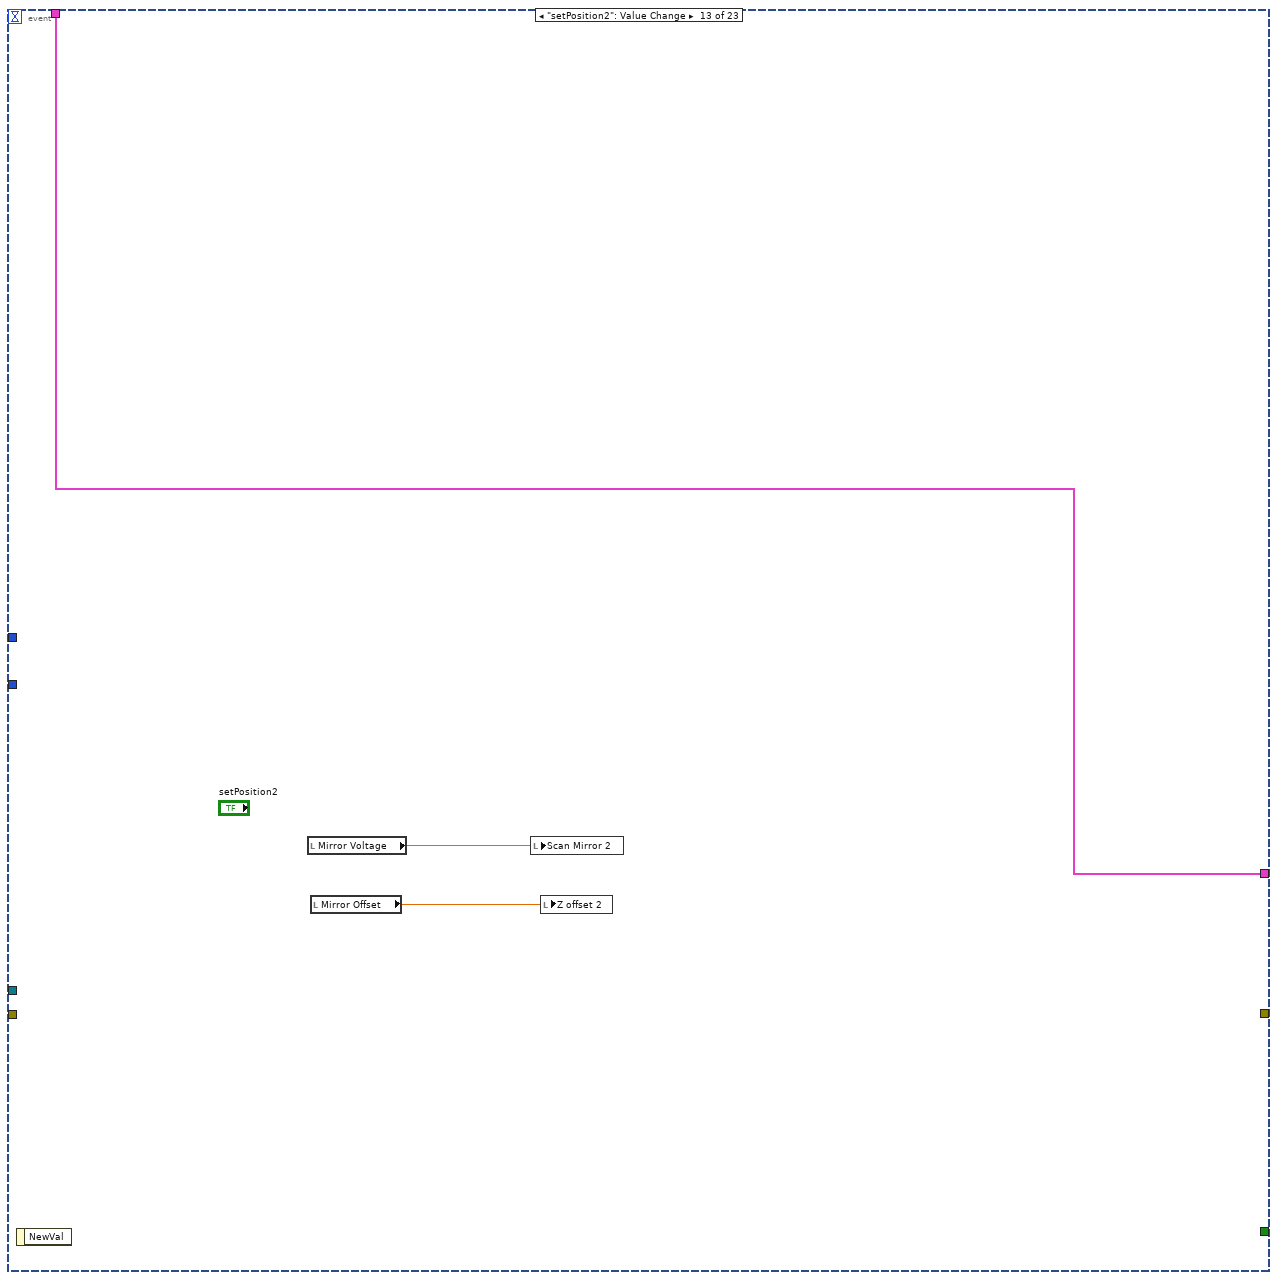
[diagram p20: hidden frame]
diagram:
  w3 = ""  # data (can be any type)
  # "PINOUT\n\nPCIe-6323\n\nConnector 1\n21 - AO1 - piezo\n22 - AO0 - scan (xy) mirror\n54 - AO GND\n55 - AO GND\n\n52 - P0.0 - AOTF  Visible Laser\n51 - P0.5 - AOTF Two-Photon Laser\n17 - P0.1 - Camera exposure\n\nConnector 2\n22 - AO2 - z mirror\n54 - AO GND\n55 - AO GND\n\n-----------------------------------\n\nPCI-6221\n12 - AO1 - tunable lens 1\n30 - AO2 - tunable lens 2\n11 - AO GND\n31 - AO GND"
  # "Releasing the queue stops the consumer loop(s)."
  # "This template is for the Producer/Consumer design pattern."
  n1 = Obtain Queue(element data type=w3) -> (queue out=w1:refnum<queue>, error out=w5:errorcluster)  [unwired: 4 in, 1 out]
  n2 = while {
    shift-right: [w14] -> w4
    shift-left: w5 -> [w17]
    tunnel: w1 -> [w18]
    shift-right: [-1] -> _
    shift-left: 0 -> [w12]
    stop <- w15 stop-if-true
    # "This loop is the producer loop."
    n3 = local read "Microscope Settings"() -> (w10:T10[])
    n4 = event shown="[2] \"Mode\": Value Change" {
      selector: _ -> [_ _ _ _ _ _ _ _ _ _ _ _ _ _ _ _ _ _ _ _ _ _ _]
      dyn-events: _ -> [_ _ _ _ _ _ _ _ _ _ _ _ _ _ _ _ _ _ _ _ _ _ _]
      timeout: w12 -> [_ _ _ _ _ _ _ _ _ _ _ _ _ _ _ _ _ _ _ _ _ _ _]
      tunnel: w18 -> [w27 _ w34 w69 w75 w83 w90 _ _ _ _ _ _ _ _ _ _ _ _ _ _ _ _]
      tunnel: w17 -> [w26 w30 w33 w68 w74 w82 w89 _ _ _ _ _ _ _ _ _ _ _ _ _ _ _ _]
      tunnel: [w25 w30 w32 w67 w73 w81 w88 _ _ _ _ _ _ _ _ _ _ _ _ _ _ _ _] -> w14
      tunnel: [_ "exit" _ _ _ _ _ _ _ _ _ _ _ _ _ _ _ _ _ _ _ _ _] -> w16
      tunnel: [w23 w29 w31 w65 w72 w80 w87 _ w120 w121 w123 w125 w128 w131 w133 w135 w137 w140 w170 w176 w212 w217 w240] -> w7
      tunnel: w10 -> [w23 w29 w31 w65 w72 w80 w87 _ w120 w121 w123 w125 w128 w131 w133 w135 w137 w140 w169 w175 w212 w218 w240]
      tunnel: "Z Mirror Control" -> [_ _ _ _ _ _ _ w91 w109 _ _ _ _ _ _ _ _ _ _ _ _ _ _]
      tunnel: "Apply ex/det correction" -> [_ _ _ _ _ _ _ _ w108 _ _ _ _ _ _ _ _ _ w146 _ _ _ _]
      event Timeout {
        w22 = T15."Enabled" ("Disabled")
        w20 = T15."Disabled and Grayed Out" ("Disabled")
        n5 = event-data() -> ()  [unwired: 1 in, 1 out]
        n6 = property on="Mode" class="Enum (strict)"("Value"=T1."Manual" ("Mode")) -> ()  [unwired: 2 in, 2 out]
        n7 = property on="Scan Mirror 2" class="DigNum (strict)"("DisabledEnum"=w22) -> ()  [unwired: 2 in, 2 out]
        n8 = property on="Scan Mirror 1" class="DigNum (strict)"("DisabledEnum"=w22) -> ()  [unwired: 2 in, 2 out]
        n9 = property on="Z offset 2" class="DigNum (strict)"("DisabledEnum"=w22) -> ()  [unwired: 2 in, 2 out]
        n10 = property on="Z offset 1" class="DigNum (strict)"("DisabledEnum"=w22) -> ()  [unwired: 2 in, 2 out]
        n11 = property on="Sample Rate (kHz)" class="DigNum (strict)"("DisabledEnum"=w20) -> ()  [unwired: 2 in, 2 out]
        n12 = Enqueue Element(queue=w27, element="manual", error in (no error)=w26) -> (error out=w25:errorcluster)  [unwired: 1 in, 2 out]
        n13 = property on="Piezo Position (µm)" class="Slide (strict)"("DisabledEnum"=w22) -> ()  [unwired: 2 in, 2 out]
        n14 = property on="Mirror Voltage" class="Slide (strict)"("DisabledEnum"=w22) -> ()  [unwired: 2 in, 2 out]
        n15 = property on="Z Mirror Gain" class="Slide (strict)"("DisabledEnum"=w22) -> ()  [unwired: 2 in, 2 out]
        n16 = property on="Mirror Offset" class="Slide (strict)"("DisabledEnum"=w22) -> ()  [unwired: 2 in, 2 out]
        n17 = property on="Lens 2" class="Slide (strict)"("DisabledEnum"=w22) -> ()  [unwired: 2 in, 2 out]
        n18 = property on="Lens 1" class="Slide (strict)"("DisabledEnum"=w22) -> ()  [unwired: 2 in, 2 out]
        n19 = property on="Sweep Interval (µS)" class="DigNum (strict)"("DisabledEnum"=w20) -> ()  [unwired: 2 in, 2 out]
        n20 = property on="Sweep Time (µS)" class="DigNum (strict)"("DisabledEnum"=w20) -> ()  [unwired: 2 in, 2 out]
        n21 = property on="MaxScanMirror" class="DigNum (strict)"("DisabledEnum"=w22) -> ()  [unwired: 2 in, 2 out]
        n22 = property on="@ max Z" class="DigNum (strict)"("DisabledEnum"=w22) -> ()  [unwired: 2 in, 2 out]
        n23 = property on="@ min Z" class="DigNum (strict)"("DisabledEnum"=w22) -> ()  [unwired: 2 in, 2 out]
        n24 = property on="Amplitude" class="DigNum (strict)"("DisabledEnum"=w20) -> ()  [unwired: 2 in, 2 out]
        n25 = property on="MinScanMirror" class="DigNum (strict)"("DisabledEnum"=w22) -> ()  [unwired: 2 in, 2 out]
        n26 = property on="set@maxZ" class="Bool"("DisabledEnum"=w22) -> ()  [unwired: 2 in, 2 out]
        n27 = property on="PiezoStartMicrometres" class="DigNum (strict)"("DisabledEnum"=w22) -> ()  [unwired: 2 in, 2 out]
        n28 = property on="set@minZ" class="Bool"("DisabledEnum"=w22) -> ()  [unwired: 2 in, 2 out]
        n29 = property on="PiezoEndMicrometres" class="DigNum (strict)"("DisabledEnum"=w22) -> ()  [unwired: 2 in, 2 out]
        n30 = property on="Z Mirror Control" class="Enum (strict)"("Value"=enum16{"manual", "automatic"}."manual") -> ()  [unwired: 2 in, 2 out]
        n31 = property on="Offset" class="DigNum (strict)"("DisabledEnum"=w20) -> ()  [unwired: 2 in, 2 out]
        n32 = property on="Phase Shift (µS)" class="Slide (strict)"("DisabledEnum"=w20) -> ()  [unwired: 2 in, 2 out]
        n33 = property on="setPiezoEnd" class="Bool"("DisabledEnum"=w22) -> ()  [unwired: 2 in, 2 out]
        n34 = property on="setPiezoStart" class="Bool"("DisabledEnum"=w22) -> ()  [unwired: 2 in, 2 out]
        n35 = property on="setPosition1" class="Bool"("DisabledEnum"=w22) -> ()  [unwired: 2 in, 2 out]
        n36 = property on="setPosition2" class="Bool"("DisabledEnum"=w22) -> ()  [unwired: 2 in, 2 out]
        n37 = property on="StopSinglePlaneScan" class="Bool"("DisabledEnum"=w20) -> ()  [unwired: 2 in, 2 out]
        n38 = property on="setScanMirrorMax" class="Bool"("DisabledEnum"=w22) -> ()  [unwired: 2 in, 2 out]
        n39 = property on="setScanMirrorMin" class="Bool"("DisabledEnum"=w22) -> ()  [unwired: 2 in, 2 out]
        n40 = property on="Time Interval  Between Repeats (µS)" class="DigNum (strict)"("DisabledEnum"=w20) -> ()  [unwired: 2 in, 2 out]
        n41 = property on="Number of Repetitions" class="DigNum (strict)"("DisabledEnum"=w20) -> ()  [unwired: 2 in, 2 out]
        n42 = property on="StartSinglePlaneScan" class="Bool"("DisabledEnum"=w20) -> ()  [unwired: 2 in, 2 out]
        n43 = property on="Apply ex/det correction" class="Enum (strict)"("DisabledEnum"=w20) -> ()  [unwired: 2 in, 2 out]
        n44 = property on="addMicroscopeSettings" class="Bool"("DisabledEnum"=w22) -> ()  [unwired: 2 in, 2 out]
        n45 = property on="deleteCurrentMicroscopeSettings" class="Bool"("DisabledEnum"=w22) -> ()  [unwired: 2 in, 2 out]
        n46 = property on="applyCurrentMicroscopeSettings" class="Bool"("DisabledEnum"=w22) -> ()  [unwired: 2 in, 2 out]
        n47 = property on="loadMicroscopeSettings" class="Bool"("DisabledEnum"=w22) -> ()  [unwired: 2 in, 2 out]
        n48 = property on="saveMicroscopeSettings" class="Bool"("DisabledEnum"=w22) -> ()  [unwired: 2 in, 2 out]
        n49 = property on="Laser" class="Enum (strict)"("DisabledEnum"=w22) -> ()  [unwired: 2 in, 2 out]
        n50 = property on="StartMultiDScan" class="Bool"("DisabledEnum"=w20) -> ()  [unwired: 2 in, 2 out]
        n51 = property on="Adjusted Scan Mirror Voltage" class="DigNum (strict)"("DisabledEnum"=w22) -> ()  [unwired: 2 in, 2 out]
        n52 = property on="Z Mirror Voltage" class="DigNum (strict)"("DisabledEnum"=w22) -> ()  [unwired: 2 in, 2 out]
        n53 = property on="StopMultiDScan" class="Bool"("DisabledEnum"=w20) -> ()  [unwired: 2 in, 2 out]
        n54 = property on="Z Mirror Control" class="Enum (strict)"("DisabledEnum"=w22) -> ()  [unwired: 2 in, 2 out]
      }
      event "exit": Value Change {
        n55 = event-data() -> ()  [unwired: 1 in, 1 out]
        n56 = shared-variable ".\\SharedVariables.lvlib\\StopSinglePlaneScan"("exit") -> ()  [unwired: 1 in, 1 out]
        n57 = shared-variable ".\\SharedVariables.lvlib\\StopScanMirrorManualControl"("exit") -> ()  [unwired: 1 in, 1 out]
        n58 = shared-variable ".\\SharedVariables.lvlib\\StopMultiDScan"("exit") -> ()  [unwired: 1 in, 1 out]
      }
      event "Mode": Value Change {
        n59 = event-data() -> ()  [unwired: 1 in, 1 out]
        n60 = case shown="\"Multi-Dimensional Scan\"" "Mode" {
          tunnel: w34 -> [w42 w53 w60]
          tunnel: w33 -> [w41 w52 w59]
          tunnel: [w40 w51 w58] -> w32
          frame "Manual", Default {
            w36 = T15."Enabled" ("Disabled")
            w39 = T15."Disabled and Grayed Out" ("Disabled")
            n61 = property on="Z Mirror Control" class="Enum (strict)"("Value"=enum16{"manual", "automatic"}."manual" ("Z Mirror Control")) -> ()  [unwired: 2 in, 2 out]
            n62 = property on="Scan Mirror 2" class="DigNum (strict)"("DisabledEnum"=w36) -> ()  [unwired: 2 in, 2 out]
            n63 = property on="Scan Mirror 1" class="DigNum (strict)"("DisabledEnum"=w36) -> ()  [unwired: 2 in, 2 out]
            n64 = property on="Z offset 2" class="DigNum (strict)"("DisabledEnum"=w36) -> ()  [unwired: 2 in, 2 out]
            n65 = property on="Z offset 1" class="DigNum (strict)"("DisabledEnum"=w36) -> ()  [unwired: 2 in, 2 out]
            n66 = property on="Sample Rate (kHz)" class="DigNum (strict)"("DisabledEnum"=w39) -> ()  [unwired: 2 in, 2 out]
            n67 = Enqueue Element(queue=w42, element="manual", error in (no error)=w41) -> (error out=w40:errorcluster)  [unwired: 1 in, 2 out]
            n68 = property on="Piezo Position (µm)" class="Slide (strict)"("DisabledEnum"=w36) -> ()  [unwired: 2 in, 2 out]
            n69 = property on="Mirror Voltage" class="Slide (strict)"("DisabledEnum"=w36) -> ()  [unwired: 2 in, 2 out]
            n70 = property on="Mirror Offset" class="Slide (strict)"("DisabledEnum"=w36) -> ()  [unwired: 2 in, 2 out]
            n71 = property on="Z Mirror Gain" class="Slide (strict)"("DisabledEnum"=w36) -> ()  [unwired: 2 in, 2 out]
            n72 = property on="Lens 2" class="Slide (strict)"("DisabledEnum"=w36) -> ()  [unwired: 2 in, 2 out]
            n73 = property on="Lens 1" class="Slide (strict)"("DisabledEnum"=w36) -> ()  [unwired: 2 in, 2 out]
            n74 = property on="Filter Wheel Position" class="DigNum (strict)"("DisabledEnum"=w36) -> ()  [unwired: 2 in, 2 out]
            n75 = property on="Sweep Time (µS)" class="DigNum (strict)"("DisabledEnum"=w39) -> ()  [unwired: 2 in, 2 out]
            n76 = shared-variable ".\\SharedVariables.lvlib\\StopSinglePlaneScan"(TRUE ("StopSinglePlaneScan")) -> ()  [unwired: 1 in, 1 out]
            n77 = property on="Phase Shift (µS)" class="Slide (strict)"("DisabledEnum"=w39) -> ()  [unwired: 2 in, 2 out]
            n78 = shared-variable ".\\SharedVariables.lvlib\\StopMultiDScan"(TRUE ("StopMultiDScan")) -> ()  [unwired: 1 in, 1 out]
            n79 = property on="Sweep Interval (µS)" class="DigNum (strict)"("DisabledEnum"=w39) -> ()  [unwired: 2 in, 2 out]
            n80 = property on="MaxScanMirror" class="DigNum (strict)"("DisabledEnum"=w36) -> ()  [unwired: 2 in, 2 out]
            n81 = property on="@ max Z" class="DigNum (strict)"("DisabledEnum"=w36) -> ()  [unwired: 2 in, 2 out]
            n82 = property on="@ min Z" class="DigNum (strict)"("DisabledEnum"=w36) -> ()  [unwired: 2 in, 2 out]
            n83 = property on="Amplitude" class="DigNum (strict)"("DisabledEnum"=w39) -> ()  [unwired: 2 in, 2 out]
            n84 = property on="MinScanMirror" class="DigNum (strict)"("DisabledEnum"=w36) -> ()  [unwired: 2 in, 2 out]
            n85 = property on="set@maxZ" class="Bool"("DisabledEnum"=w36) -> ()  [unwired: 2 in, 2 out]
            n86 = property on="PiezoEndMicrometres" class="DigNum (strict)"("DisabledEnum"=w36) -> ()  [unwired: 2 in, 2 out]
            n87 = property on="set@minZ" class="Bool"("DisabledEnum"=w36) -> ()  [unwired: 2 in, 2 out]
            n88 = property on="PiezoStartMicrometres" class="DigNum (strict)"("DisabledEnum"=w36) -> ()  [unwired: 2 in, 2 out]
            n89 = property on="Offset" class="DigNum (strict)"("DisabledEnum"=w39) -> ()  [unwired: 2 in, 2 out]
            n90 = property on="setPiezoEnd" class="Bool"("DisabledEnum"=w36) -> ()  [unwired: 2 in, 2 out]
            n91 = property on="setPiezoStart" class="Bool"("DisabledEnum"=w36) -> ()  [unwired: 2 in, 2 out]
            n92 = property on="setPosition1" class="Bool"("DisabledEnum"=w36) -> ()  [unwired: 2 in, 2 out]
            n93 = property on="setPosition2" class="Bool"("DisabledEnum"=w36) -> ()  [unwired: 2 in, 2 out]
            n94 = property on="StopSinglePlaneScan" class="Bool"("DisabledEnum"=w39) -> ()  [unwired: 2 in, 2 out]
            n95 = property on="setScanMirrorMax" class="Bool"("DisabledEnum"=w36) -> ()  [unwired: 2 in, 2 out]
            n96 = property on="setScanMirrorMin" class="Bool"("DisabledEnum"=w36) -> ()  [unwired: 2 in, 2 out]
            n97 = property on="Apply ex/det correction" class="Enum (strict)"("DisabledEnum"=w39) -> ()  [unwired: 2 in, 2 out]
            n98 = property on="StartSinglePlaneScan" class="Bool"("DisabledEnum"=w39) -> ()  [unwired: 2 in, 2 out]
            n99 = property on="addMicroscopeSettings" class="Bool"("DisabledEnum"=w36) -> ()  [unwired: 2 in, 2 out]
            n100 = property on="deleteCurrentMicroscopeSettings" class="Bool"("DisabledEnum"=w36) -> ()  [unwired: 2 in, 2 out]
            n101 = property on="applyCurrentMicroscopeSettings" class="Bool"("DisabledEnum"=w36) -> ()  [unwired: 2 in, 2 out]
            n102 = property on="loadMicroscopeSettings" class="Bool"("DisabledEnum"=w36) -> ()  [unwired: 2 in, 2 out]
            n103 = property on="saveMicroscopeSettings" class="Bool"("DisabledEnum"=w36) -> ()  [unwired: 2 in, 2 out]
            n104 = property on="Laser" class="Enum (strict)"("DisabledEnum"=w36) -> ()  [unwired: 2 in, 2 out]
            n105 = property on="Adjusted Scan Mirror Voltage" class="DigNum (strict)"("DisabledEnum"=w36) -> ()  [unwired: 2 in, 2 out]
            n106 = property on="Z Mirror Voltage" class="DigNum (strict)"("DisabledEnum"=w36) -> ()  [unwired: 2 in, 2 out]
            n107 = property on="Number of Z Slices" class="DigNum (strict)"("DisabledEnum"=w36) -> ()  [unwired: 2 in, 2 out]
            n108 = property on="Z Mirror Control" class="Enum (strict)"("DisabledEnum"=w36) -> ()  [unwired: 2 in, 2 out]
            n109 = property on="StartMultiDScan" class="Bool"("DisabledEnum"=w39) -> ()  [unwired: 2 in, 2 out]
            n110 = property on="StopMultiDScan" class="Bool"("DisabledEnum"=w39) -> ()  [unwired: 2 in, 2 out]
            n111 = property on="Number of Repetitions" class="DigNum (strict)"("DisabledEnum"=w39) -> ()  [unwired: 2 in, 2 out]
            n112 = property on="Time Interval  Between Stacks (µS)" class="DigNum (strict)"("DisabledEnum"=w39) -> ()  [unwired: 2 in, 2 out]
          }
          frame "Single Plane Scan" {
            w54 = T15."Disabled and Grayed Out" ("Disabled")
            w45 = T15."Enabled" ("Disabled")
            n113 = local read "MaxScanMirror"() -> (w48:T3)
            n114 = local read "MinScanMirror"() -> (w47:T3)
            n115 = property on="Scan Mirror 2" class="DigNum (strict)"("DisabledEnum"=w54) -> ()  [unwired: 2 in, 2 out]
            n116 = property on="Scan Mirror 1" class="DigNum (strict)"("DisabledEnum"=w54) -> ()  [unwired: 2 in, 2 out]
            n117 = property on="Z offset 2" class="DigNum (strict)"("DisabledEnum"=w54) -> ()  [unwired: 2 in, 2 out]
            n118 = property on="Z offset 1" class="DigNum (strict)"("DisabledEnum"=w54) -> ()  [unwired: 2 in, 2 out]
            n119 = property on="Phase Shift (µS)" class="Slide (strict)"("DisabledEnum"=w45) -> ()  [unwired: 2 in, 2 out]
            n120 = Subtract(x=w48, y=w47) -> (x-y=w46:T3)
            n121 = property on="Piezo Position (µm)" class="Slide (strict)"("DisabledEnum"=w54) -> ()  [unwired: 2 in, 2 out]
            n122 = property on="Mirror Voltage" class="Slide (strict)"("DisabledEnum"=w54) -> ()  [unwired: 2 in, 2 out]
            n123 = property on="Mirror Offset" class="Slide (strict)"("DisabledEnum"=w54) -> ()  [unwired: 2 in, 2 out]
            n124 = property on="Z Mirror Gain" class="Slide (strict)"("DisabledEnum"=w54) -> ()  [unwired: 2 in, 2 out]
            n125 = property on="Lens 2" class="Slide (strict)"("DisabledEnum"=w54) -> ()  [unwired: 2 in, 2 out]
            n126 = property on="Lens 1" class="Slide (strict)"("DisabledEnum"=w54) -> ()  [unwired: 2 in, 2 out]
            n127 = property on="Amplitude" class="DigNum (strict)"("DisabledEnum"=w45) -> ()  [unwired: 2 in, 2 out]
            n128 = property on="Sample Rate (kHz)" class="DigNum (strict)"("DisabledEnum"=w45) -> ()  [unwired: 2 in, 2 out]
            n129 = local write "Amplitude"(w46) -> ()
            n130 = local write "Offset"(w47) -> ()
            n131 = Flush Queue(queue=w53, error in (no error)=w52) -> (error out=w51:errorcluster)  [unwired: 2 out]
            n132 = property on="Sweep Interval (µS)" class="DigNum (strict)"("DisabledEnum"=w45) -> ()  [unwired: 2 in, 2 out]
            n133 = property on="MaxScanMirror" class="DigNum (strict)"("DisabledEnum"=w54) -> ()  [unwired: 2 in, 2 out]
            n134 = property on="@ max Z" class="DigNum (strict)"("DisabledEnum"=w54) -> ()  [unwired: 2 in, 2 out]
            n135 = property on="@ min Z" class="DigNum (strict)"("DisabledEnum"=w54) -> ()  [unwired: 2 in, 2 out]
            n136 = property on="Sweep Time (µS)" class="DigNum (strict)"("DisabledEnum"=w45) -> ()  [unwired: 2 in, 2 out]
            n137 = property on="MinScanMirror" class="DigNum (strict)"("DisabledEnum"=w54) -> ()  [unwired: 2 in, 2 out]
            n138 = property on="set@maxZ" class="Bool"("DisabledEnum"=w54) -> ()  [unwired: 2 in, 2 out]
            n139 = property on="PiezoEndMicrometres" class="DigNum (strict)"("DisabledEnum"=w54) -> ()  [unwired: 2 in, 2 out]
            n140 = property on="set@minZ" class="Bool"("DisabledEnum"=w54) -> ()  [unwired: 2 in, 2 out]
            n141 = property on="PiezoStartMicrometres" class="DigNum (strict)"("DisabledEnum"=w54) -> ()  [unwired: 2 in, 2 out]
            n142 = property on="Filter Wheel Position" class="DigNum (strict)"("DisabledEnum"=w45) -> ()  [unwired: 2 in, 2 out]
            n143 = shared-variable ".\\SharedVariables.lvlib\\StopScanMirrorManualControl"(TRUE ("StopScanMirrorManualControl")) -> ()  [unwired: 1 in, 1 out]
            n144 = property on="Offset" class="DigNum (strict)"("DisabledEnum"=w45) -> ()  [unwired: 2 in, 2 out]
            n145 = shared-variable ".\\SharedVariables.lvlib\\StopMultiDScan"(TRUE ("StopMultiDScan")) -> ()  [unwired: 1 in, 1 out]
            n146 = property on="StopSinglePlaneScan" class="Bool"("DisabledEnum"=w45) -> ()  [unwired: 2 in, 2 out]
            n147 = property on="setPiezoEnd" class="Bool"("DisabledEnum"=w54) -> ()  [unwired: 2 in, 2 out]
            n148 = property on="setPiezoStart" class="Bool"("DisabledEnum"=w54) -> ()  [unwired: 2 in, 2 out]
            n149 = property on="setPosition1" class="Bool"("DisabledEnum"=w54) -> ()  [unwired: 2 in, 2 out]
            n150 = property on="setPosition2" class="Bool"("DisabledEnum"=w54) -> ()  [unwired: 2 in, 2 out]
            n151 = property on="setScanMirrorMax" class="Bool"("DisabledEnum"=w54) -> ()  [unwired: 2 in, 2 out]
            n152 = property on="setScanMirrorMin" class="Bool"("DisabledEnum"=w54) -> ()  [unwired: 2 in, 2 out]
            n153 = property on="StartSinglePlaneScan" class="Bool"("DisabledEnum"=w45) -> ()  [unwired: 2 in, 2 out]
            n154 = property on="addMicroscopeSettings" class="Bool"("DisabledEnum"=w54) -> ()  [unwired: 2 in, 2 out]
            n155 = property on="deleteCurrentMicroscopeSettings" class="Bool"("DisabledEnum"=w54) -> ()  [unwired: 2 in, 2 out]
            n156 = property on="applyCurrentMicroscopeSettings" class="Bool"("DisabledEnum"=w54) -> ()  [unwired: 2 in, 2 out]
            n157 = property on="loadMicroscopeSettings" class="Bool"("DisabledEnum"=w54) -> ()  [unwired: 2 in, 2 out]
            n158 = property on="saveMicroscopeSettings" class="Bool"("DisabledEnum"=w54) -> ()  [unwired: 2 in, 2 out]
            n159 = property on="Laser" class="Enum (strict)"("DisabledEnum"=w54) -> ()  [unwired: 2 in, 2 out]
            n160 = property on="Number of Z Slices" class="DigNum (strict)"("DisabledEnum"=w54) -> ()  [unwired: 2 in, 2 out]
            n161 = property on="StartMultiDScan" class="Bool"("DisabledEnum"=w54) -> ()  [unwired: 2 in, 2 out]
            n162 = property on="Number of Repetitions" class="DigNum (strict)"("DisabledEnum"=w54) -> ()  [unwired: 2 in, 2 out]
            n163 = property on="Apply ex/det correction" class="Enum (strict)"("DisabledEnum"=w54) -> ()  [unwired: 2 in, 2 out]
            n164 = property on="Adjusted Scan Mirror Voltage" class="DigNum (strict)"("DisabledEnum"=w54) -> ()  [unwired: 2 in, 2 out]
            n165 = property on="Z Mirror Voltage" class="DigNum (strict)"("DisabledEnum"=w54) -> ()  [unwired: 2 in, 2 out]
            n166 = property on="Z Mirror Control" class="Enum (strict)"("DisabledEnum"=w54) -> ()  [unwired: 2 in, 2 out]
            n167 = property on="StopMultiDScan" class="Bool"("DisabledEnum"=w54) -> ()  [unwired: 2 in, 2 out]
            n168 = property on="Time Interval  Between Stacks (µS)" class="DigNum (strict)"("DisabledEnum"=w54) -> ()  [unwired: 2 in, 2 out]
          }
          frame "Multi-Dimensional Scan" {
            w62 = T15."Enabled" ("Disabled")
            w56 = T15."Disabled and Grayed Out" ("Disabled")
            n169 = property on="Scan Mirror 1" class="DigNum (strict)"("DisabledEnum"=w56) -> ()  [unwired: 2 in, 2 out]
            n170 = property on="Scan Mirror 2" class="DigNum (strict)"("DisabledEnum"=w56) -> ()  [unwired: 2 in, 2 out]
            n171 = property on="Z offset 1" class="DigNum (strict)"("DisabledEnum"=w56) -> ()  [unwired: 2 in, 2 out]
            n172 = property on="Z offset 2" class="DigNum (strict)"("DisabledEnum"=w56) -> ()  [unwired: 2 in, 2 out]
            n173 = Flush Queue(queue=w60, error in (no error)=w59) -> (error out=w58:errorcluster)  [unwired: 2 out]
            n174 = call "DAQ Assistant"("data"=digitalwaveform[] [{"t0"=timestamp(0 s since 1904-01-01), "dt"=0.0, "Y"={"transitions"=[0, 1, 2, 3, 4], "data"=[[0], [0], [0], [0], [0]]}, "error"={"status"=FALSE, "code"=37421928, "source"=""}}, {"t0"=timestamp(0 s since 1904-01-01), "dt"=0.0, "Y"={"transitions"=[0, 1, 2, 3, 4], "data"=[[0], [0], [0], [0], [0]]}, "error"={"status"=FALSE, "code"=37421928, "source"=""}}]) -> ()  [unwired: 17 in, 2 out]
            n175 = property on="Mirror Voltage" class="Slide (strict)"("DisabledEnum"=w56) -> ()  [unwired: 2 in, 2 out]
            n176 = property on="Piezo Position (µm)" class="Slide (strict)"("DisabledEnum"=w56) -> ()  [unwired: 2 in, 2 out]
            n177 = property on="Mirror Offset" class="Slide (strict)"("DisabledEnum"=w56) -> ()  [unwired: 2 in, 2 out]
            n178 = property on="Z Mirror Gain" class="Slide (strict)"("DisabledEnum"=w56) -> ()  [unwired: 2 in, 2 out]
            n179 = property on="Lens 1" class="Slide (strict)"("DisabledEnum"=w56) -> ()  [unwired: 2 in, 2 out]
            n180 = property on="Lens 2" class="Slide (strict)"("DisabledEnum"=w56) -> ()  [unwired: 2 in, 2 out]
            n181 = shared-variable ".\\SharedVariables.lvlib\\StopScanMirrorManualControl"(TRUE ("StopScanMirrorManualControl")) -> ()  [unwired: 1 in, 1 out]
            n182 = property on="Sample Rate (kHz)" class="DigNum (strict)"("DisabledEnum"=w56) -> ()  [unwired: 2 in, 2 out]
            n183 = property on="Phase Shift (µS)" class="Slide (strict)"("DisabledEnum"=w56) -> ()  [unwired: 2 in, 2 out]
            n184 = property on="Filter Wheel Position" class="DigNum (strict)"("DisabledEnum"=w56) -> ()  [unwired: 2 in, 2 out]
            n185 = property on="MaxScanMirror" class="DigNum (strict)"("DisabledEnum"=w56) -> ()  [unwired: 2 in, 2 out]
            n186 = property on="@ min Z" class="DigNum (strict)"("DisabledEnum"=w56) -> ()  [unwired: 2 in, 2 out]
            n187 = property on="MinScanMirror" class="DigNum (strict)"("DisabledEnum"=w56) -> ()  [unwired: 2 in, 2 out]
            n188 = property on="@ max Z" class="DigNum (strict)"("DisabledEnum"=w56) -> ()  [unwired: 2 in, 2 out]
            n189 = property on="PiezoStartMicrometres" class="DigNum (strict)"("DisabledEnum"=w56) -> ()  [unwired: 2 in, 2 out]
            n190 = property on="PiezoEndMicrometres" class="DigNum (strict)"("DisabledEnum"=w56) -> ()  [unwired: 2 in, 2 out]
            n191 = property on="set@maxZ" class="Bool"("DisabledEnum"=w56) -> ()  [unwired: 2 in, 2 out]
            n192 = property on="set@minZ" class="Bool"("DisabledEnum"=w56) -> ()  [unwired: 2 in, 2 out]
            n193 = shared-variable ".\\SharedVariables.lvlib\\StopSinglePlaneScan"(TRUE ("StopSinglePlaneScan")) -> ()  [unwired: 1 in, 1 out]
            n194 = property on="Sweep Interval (µS)" class="DigNum (strict)"("DisabledEnum"=w56) -> ()  [unwired: 2 in, 2 out]
            n195 = property on="Sweep Time (µS)" class="DigNum (strict)"("DisabledEnum"=w56) -> ()  [unwired: 2 in, 2 out]
            n196 = property on="setPiezoEnd" class="Bool"("DisabledEnum"=w56) -> ()  [unwired: 2 in, 2 out]
            n197 = property on="setPiezoStart" class="Bool"("DisabledEnum"=w56) -> ()  [unwired: 2 in, 2 out]
            n198 = property on="setPosition1" class="Bool"("DisabledEnum"=w56) -> ()  [unwired: 2 in, 2 out]
            n199 = property on="setPosition2" class="Bool"("DisabledEnum"=w56) -> ()  [unwired: 2 in, 2 out]
            n200 = property on="setScanMirrorMax" class="Bool"("DisabledEnum"=w56) -> ()  [unwired: 2 in, 2 out]
            n201 = property on="setScanMirrorMin" class="Bool"("DisabledEnum"=w56) -> ()  [unwired: 2 in, 2 out]
            n202 = property on="Offset" class="DigNum (strict)"("DisabledEnum"=w56) -> ()  [unwired: 2 in, 2 out]
            n203 = property on="Amplitude" class="DigNum (strict)"("DisabledEnum"=w56) -> ()  [unwired: 2 in, 2 out]
            n204 = property on="addMicroscopeSettings" class="Bool"("DisabledEnum"=w56) -> ()  [unwired: 2 in, 2 out]
            n205 = property on="applyCurrentMicroscopeSettings" class="Bool"("DisabledEnum"=w56) -> ()  [unwired: 2 in, 2 out]
            n206 = property on="Z Mirror Control" class="Enum (strict)"("DisabledEnum"=w56) -> ()  [unwired: 2 in, 2 out]
            n207 = property on="Laser" class="Enum (strict)"("DisabledEnum"=w56) -> ()  [unwired: 2 in, 2 out]
            n208 = property on="Apply ex/det correction" class="Enum (strict)"("DisabledEnum"=w56) -> ()  [unwired: 2 in, 2 out]
            n209 = property on="Adjusted Scan Mirror Voltage" class="DigNum (strict)"("DisabledEnum"=w56) -> ()  [unwired: 2 in, 2 out]
            n210 = property on="Number of Z Slices" class="DigNum (strict)"("DisabledEnum"=w56) -> ()  [unwired: 2 in, 2 out]
            n211 = property on="Mirror Voltage" class="Slide (strict)"("DisabledEnum"=w56) -> ()  [unwired: 2 in, 2 out]
            n212 = property on="StartSinglePlaneScan" class="Bool"("DisabledEnum"=w56) -> ()  [unwired: 2 in, 2 out]
            n213 = property on="StopSinglePlaneScan" class="Bool"("DisabledEnum"=w56) -> ()  [unwired: 2 in, 2 out]
            n214 = property on="deleteCurrentMicroscopeSettings" class="Bool"("DisabledEnum"=w62) -> ()  [unwired: 2 in, 2 out]
            n215 = property on="loadMicroscopeSettings" class="Bool"("DisabledEnum"=w62) -> ()  [unwired: 2 in, 2 out]
            n216 = property on="saveMicroscopeSettings" class="Bool"("DisabledEnum"=w62) -> ()  [unwired: 2 in, 2 out]
            n217 = property on="StartMultiDScan" class="Bool"("DisabledEnum"=w62) -> ()  [unwired: 2 in, 2 out]
            n218 = property on="StopMultiDScan" class="Bool"("DisabledEnum"=w62) -> ()  [unwired: 2 in, 2 out]
            n219 = property on="Number of Repetitions" class="DigNum (strict)"("DisabledEnum"=w62) -> ()  [unwired: 2 in, 2 out]
            n220 = property on="Time Interval  Between Stacks (µS)" class="DigNum (strict)"("DisabledEnum"=w62) -> ()  [unwired: 2 in, 2 out]
          }
        }
      }
      event "StartSinglePlaneScan": Value Change {
        # "Generate the data here."
        n221 = event-data() -> ()  [unwired: 1 in, 1 out]
        n222 = Enqueue Element(queue=w69, element="SinglePlaneScan", error in (no error)=w68) -> (error out=w67:errorcluster)  [unwired: 1 in, 2 out]
        n223 = property on="StopSinglePlaneScan" class="Bool"("DisabledEnum"=T15."Enabled" ("Disabled")) -> ()  [unwired: 2 in, 2 out]
        n224 = property on="StartSinglePlaneScan" class="Bool"("DisabledEnum"=T15."Disabled and Grayed Out" ("Disabled")) -> ()  [unwired: 2 in, 2 out]
      }
      event "StopSinglePlaneScan": Value Change {
        n225 = event-data() -> ()  [unwired: 1 in, 1 out]
        n226 = shared-variable ".\\SharedVariables.lvlib\\StopSinglePlaneScan"("StopSinglePlaneScan") -> ()  [unwired: 1 in, 1 out]
        n227 = Flush Queue(queue=w75, error in (no error)=w74) -> (error out=w73:errorcluster)  [unwired: 2 out]
        n228 = property on="StartSinglePlaneScan" class="Bool"("DisabledEnum"=T15."Enabled" ("Disabled")) -> ()  [unwired: 2 in, 2 out]
        n229 = property on="StopSinglePlaneScan" class="Bool"("DisabledEnum"=T15."Disabled and Grayed Out" ("Disabled")) -> ()  [unwired: 2 in, 2 out]
      }
      event "StartMultiDScan": Value Change {
        n230 = event-data() -> ()  [unwired: 1 in, 1 out]
        n231 = Enqueue Element(queue=w83, element="MultiDScan", error in (no error)=w82) -> (error out=w81:errorcluster)  [unwired: 1 in, 2 out]
        n232 = property on="StopMultiDScan" class="Bool"("DisabledEnum"=T15."Enabled" ("Disabled")) -> ()  [unwired: 2 in, 2 out]
        n233 = property on="StartMultiDScan" class="Bool"("DisabledEnum"=T15."Disabled and Grayed Out" ("Disabled")) -> ()  [unwired: 2 in, 2 out]
      }
      event "StopMultiDScan": Value Change {
        n234 = event-data() -> ()  [unwired: 1 in, 1 out]
        n235 = Flush Queue(queue=w90, error in (no error)=w89) -> (error out=w88:errorcluster)  [unwired: 2 out]
        n236 = property on="StartMultiDScan" class="Bool"("DisabledEnum"=T15."Enabled" ("Disabled")) -> ()  [unwired: 2 in, 2 out]
        n237 = property on="StopMultiDScan" class="Bool"("DisabledEnum"=T15."Disabled and Grayed Out" ("Disabled")) -> ()  [unwired: 2 in, 2 out]
        n238 = shared-variable ".\\SharedVariables.lvlib\\StopMultiDScan"(TRUE ("StopMultiDScan")) -> ()  [unwired: 1 in, 1 out]
      }
      event "Z Mirror Control": Value Change {
        n239 = event-data() -> ()  [unwired: 1 in, 1 out]
        n240 = case shown="\"manual\", Default" w91 {
          frame "manual", Default {
            w93 = T15."Disabled and Grayed Out" ("Disabled")
            n241 = property on="Mirror Offset" class="Slide (strict)"("DisabledEnum"=w93) -> ()  [unwired: 2 in, 2 out]
            n242 = property on="Z Mirror Gain" class="Slide (strict)"("DisabledEnum"=w93) -> ()  [unwired: 2 in, 2 out]
            n243 = property on="setPosition1" class="Bool"("DisabledEnum"=w93) -> ()  [unwired: 2 in, 2 out]
            n244 = property on="setPosition2" class="Bool"("DisabledEnum"=w93) -> ()  [unwired: 2 in, 2 out]
            n245 = property on="Apply ex/det correction" class="Enum (strict)"("DisabledEnum"=T15."Enabled" ("Disabled")) -> ()  [unwired: 2 in, 2 out]
          }
          frame "automatic" {
            w95 = T15."Enabled" ("Disabled")
            n246 = property on="Z Mirror Gain" class="Slide (strict)"("DisabledEnum"=w95) -> ()  [unwired: 2 in, 2 out]
            n247 = property on="Mirror Offset" class="Slide (strict)"("DisabledEnum"=w95) -> ()  [unwired: 2 in, 2 out]
            n248 = property on="setPosition1" class="Bool"("DisabledEnum"=w95) -> ()  [unwired: 2 in, 2 out]
            n249 = property on="setPosition2" class="Bool"("DisabledEnum"=w95) -> ()  [unwired: 2 in, 2 out]
            n250 = property on="Apply ex/det correction" class="Enum (strict)"("DisabledEnum"=T15."Disabled and Grayed Out" ("Disabled")) -> ()  [unwired: 2 in, 2 out]
          }
        }
      }
      event "Mirror Voltage", "Mirror Offset": Value Change {
        n251 = event-data() -> ()  [unwired: 1 in, 1 out]
        n252 = shared-variable ".\\SharedVariables.lvlib\\Laser"("Laser") -> ()  [unwired: 1 in, 1 out]
        n253 = call "mirrorCorrections.vi"("Scan Mirror Min"="MinScanMirror", "Beam@maxZ"="@ max Z", "Z Mirror Offset"="Mirror Offset", "Z Mirror Gain"="Z Mirror Gain", "Piezo Position (µm)"="Piezo Position (µm)", "Piezo Min (µm)"="PiezoStartMicrometres", "Piezo Max (µm)"="PiezoEndMicrometres", "Scan Mirror Max"="MaxScanMirror", "Scan Mirror Voltage"="Mirror Voltage", "Scan Mirror Position 2"="Scan Mirror 2", "Z Mirror Control"=w109, "Z Offset Position 2"="Z offset 2", "Apply ex/det correction"=w108) -> ("Adjusted Scan Mirror Voltage"=w107:T3, "Z Mirror Voltage"=w106:T3)  [unwired: 13 in]
        "Adjusted Scan Mirror Voltage" <- w107
        "Z Mirror Voltage" <- w106
        n254 = shared-variable ".\\SharedVariables.lvlib\\ScanMirrorVoltage"(w107) -> ()  [unwired: 1 in, 1 out]
        n255 = shared-variable ".\\SharedVariables.lvlib\\ZMirrorVoltage"(w106) -> ()  [unwired: 1 in, 1 out]
        n256 = shared-variable ".\\SharedVariables.lvlib\\PiezoMicrometres"("Piezo Position (µm)") -> ()  [unwired: 1 in, 1 out]
        n257 = In Range and Coerce(upper limit=T5 3.0, x="Lens 1", lower limit=T5 0.0) -> (coerced(x)=w103:T5)  [unwired: 1 out]
        n258 = In Range and Coerce(upper limit=T5 3.0, x="Lens 2", lower limit=T5 0.0) -> (coerced(x)=w104:T5)  [unwired: 1 out]
        n259 = shared-variable ".\\SharedVariables.lvlib\\Lens1"(w103) -> ()  [unwired: 1 in, 1 out]
        n260 = shared-variable ".\\SharedVariables.lvlib\\Lens2"(w104) -> ()  [unwired: 1 in, 1 out]
      }
      event "setScanMirrorMax": Value Change {
        n261 = event-data() -> ()  [unwired: 1 in, 1 out]
        n262 = local read "Mirror Voltage"() -> (w122:dbl)
        n263 = local write "MaxScanMirror"(w122) -> ()
      }
      event "setScanMirrorMin": Value Change {
        n264 = event-data() -> ()  [unwired: 1 in, 1 out]
        n265 = local read "Mirror Voltage"() -> (w124:dbl)
        n266 = local write "MinScanMirror"(w124) -> ()
      }
      event "setPosition1": Value Change {
        n267 = event-data() -> ()  [unwired: 1 in, 1 out]
        n268 = local read "Mirror Voltage"() -> (w127:dbl)
        n269 = local read "Mirror Offset"() -> (w126:dbl)
        n270 = local write "Z offset 1"(w126) -> ()
        n271 = local write "Scan Mirror 1"(w127) -> ()
      }
      event "setPosition2": Value Change {
        n272 = event-data() -> ()  [unwired: 1 in, 1 out]
        n273 = local read "Mirror Voltage"() -> (w130:dbl)
        n274 = local read "Mirror Offset"() -> (w129:dbl)
        n275 = local write "Scan Mirror 2"(w130) -> ()
        n276 = local write "Z offset 2"(w129) -> ()
      }
      event "setPiezoStart": Value Change {
        n277 = event-data() -> ()  [unwired: 1 in, 1 out]
        n278 = local read "Piezo Position (µm)"() -> (w132:T8)
        n279 = local write "PiezoStartMicrometres"(w132) -> ()
      }
      event "setPiezoEnd": Value Change {
        n280 = event-data() -> ()  [unwired: 1 in, 1 out]
        n281 = local read "Piezo Position (µm)"() -> (w134:T8)
        n282 = local write "PiezoEndMicrometres"(w134) -> ()
      }
      event "set@maxZ": Value Change {
        n283 = event-data() -> ()  [unwired: 1 in, 1 out]
        n284 = local read "Mirror Voltage"() -> (w136:dbl)
        n285 = local write "@ max Z"(w136) -> ()
      }
      event "set@minZ": Value Change {
        n286 = event-data() -> ()  [unwired: 1 in, 1 out]
        n287 = local read "Mirror Voltage"() -> (w138:dbl)
        n288 = local write "@ min Z"(w138) -> ()
      }
      event "Filter Wheel Position": Value Change {
        n289 = event-data() -> ()  [unwired: 1 in, 5 out]
        n290 = shared-variable "My Computer\\SharedVariables.lvlib\\COMport"() -> (w139:i32)  [unwired: 1 in, 1 out]
        n291 = call "filterWheel.vi"("serial  port"=w139, "position"="Filter Wheel Position") -> ()  [unwired: 10 in]
      }
      event "addMicroscopeSettings": Value Change {
        n292 = event-data() -> ()  [unwired: 1 in, 1 out]
        n293 = local read "MaxScanMirror"() -> (w163:T3)
        n294 = local read "MinScanMirror"() -> (w162:T3)
        n295 = local read "PiezoStartMicrometres"() -> (w151:T4)
        n296 = local read "PiezoEndMicrometres"() -> (w150:T4)
        n297 = local read "Filter Wheel Position"() -> (w147:i32)
        n298 = local read "Sweep Interval (µS)"() -> (w166:T2)
        n299 = local read "Number of Z Slices"() -> (w148:i16)
        n300 = local read "Sample Rate (kHz)"() -> (w165:i32)
        n301 = local read "Sweep Time (µS)"() -> (w167:T2)
        n302 = local read "Phase Shift (µS)"() -> (w164:i32)
        n303 = local read "Mirror Offset"() -> (w142:dbl)
        n304 = local read "Z Mirror Gain"() -> (w160:T6)
        n305 = local read "Scan Mirror 1"() -> (w159:T3)
        n306 = local read "Scan Mirror 2"() -> (w157:T3)
        n307 = local read "Z offset 1"() -> (w158:T9)
        n308 = local read "Z offset 2"() -> (w156:T9)
        n309 = local read "@ min Z"() -> (w153:T3)
        n310 = local read "@ max Z"() -> (w152:T3)
        n311 = Subtract(x=w163, y=w162) -> (x-y=w161:T3)
        n312 = local read "Lens 1"() -> (w155:T5)
        n313 = local read "Lens 2"() -> (w154:T5)
        n314 = local read "Laser"() -> (w168:T7)
        n315 = Bundle("Laser"=w168, "Sweep Time (µS)"=w167, "Sweep Interval (µS)"=w166, "Sample Rate (kHz)"=w165, "Phase Shift (µS)"=w164, "MaxScanMirror"=w163, "MinScanMirror"=w162, "MaxScanMirror"=w161, "Mirror Offset"=w142, "Z Mirror Gain"=w160, "Scan Mirror 1"=w159, "Z offset 1"=w158, "Scan Mirror 2"=w157, "Z offset 2"=w156, "Lens 1"=w155, "Lens 2"=w154, "@ min Z"=w153, "@ max Z"=w152, "PiezoStartMicrometres"=w151, "PiezoEndMicrometres"=w150, "Number of Z Slices"=w148, "Filter Wheel Position"=w147, "Apply ex/det correction"=w146) -> (w149:T18)  [unwired: 1 in]
        n316 = Index Array(array=w169, index=0) -> (element=w143:T10)
        n317 = call "Waveform_Generation2.vi"("input cluster"=w149) -> ("output cluster"=w145:T14)  [unwired: 9 in]
        n318 = Bundle By Name(cluster=w143, "Laser"=w168, "Sweep Time (µS)"=w167, "Sweep Interval (µS)"=w166, "Sample Rate (kHz)"=w165, "Camera Phase Shift (µS)"=w164, "Scan Mirror Max"=w163, "Scan Mirror Min"=w162, "Scan Mirror Amplitude"=w161, "Z Offset"=w142, "Z Gain"=w160, "Scan Mirror Position 1"=w159, "Z Offset Position 1"=w158, "Scan Mirror Position 2"=w157, "Z Offset Position 2"=w156, "Tuneable Lens 1"=w155, "Tuneable Lens 2"=w154, "Beam @ min Z"=w153, "Beam @ max Z"=w152, "Piezo Start (µm)"=w151, "Piezo End (µm)"=w150, "Number Z Slices"=w148, "Filter Wheel Position"=w147, "Apply ex/det correction"=w146, "waveforms"=w145) -> (w144:T10)
        n319 = Build Array (concatenate)(w169, w144) -> (w170:T10[])
        n320 = Array Size(array=w170) -> (size(s)=w173:i32)
        n321 = Decrement(x=w173) -> (x-1=w174:i32)
        n322 = Build Array(w174) -> (w172:i32[])
        n323 = property on="Microscope Settings" class="Arr (strict)"("Index Values"=w172) -> ()  [unwired: 2 in, 2 out]
      }
      event "deleteCurrentMicroscopeSettings": Value Change {
        n324 = event-data() -> ()  [unwired: 1 in, 1 out]
        n325 = Two Button Dialog(message="Delete current setting from array", 1:"No" ("F button name (\"Cancel\")"), 2:"Yes" ("T button name (\"OK\")")) -> (T button?=w177:bool)
        n326 = case shown="True" w177 {
          tunnel: w175 -> [w181 w186]
          tunnel: [w181 w182] -> w176
          frame False {
          }
          frame True {
            n327 = property on="Microscope Settings" class="Arr (strict)"() -> ("Index Values"=w185:u32[])  [unwired: 2 in, 2 out]
            n328 = for {
              tunnel: w185 -> [w189] mode=indexing
              tunnel: [w189] -> w184
            }
            n329 = Decrement(x=w184) -> (x-1=w187:u32)
            n330 = Build Array(w187) -> (w183:u32[])
            n331 = Delete From Array(array=w186, length=1) -> (array with subset deleted=w182:T10[])  [unwired: 1 in, 1 out]
            n332 = property on="Microscope Settings" class="Arr (strict)"("Index Values"=w183) -> ()  [unwired: 2 in, 2 out]
          }
        }
      }
      event "applyCurrentMicroscopeSettings": Value Change {
        # "Apply Current Settings"
        n333 = event-data() -> ()  [unwired: 1 in, 1 out]
        n334 = property on="Microscope Settings" class="Arr (strict)"() -> ("Index Values"=w214:u32[])  [unwired: 2 in, 2 out]
        n335 = for {
          tunnel: w214 -> [w216] mode=indexing
          tunnel: [w216] -> w215
        }
        n336 = Index Array(array=w212, index=w215) -> (element=w213:T10)
        n337 = Unbundle By Name(w213) -> ("Laser"=w211:T7, "Sweep Time (µS)"=w210:T2, "Sweep Interval (µS)"=w209:T2, "Sample Rate (kHz)"=w208:dbl, "Camera Phase Shift (µS)"=w207:T11, "Scan Mirror Max"=w206:T3, "Scan Mirror Min"=w205:T3, "Z Offset"=w191:T9, "Z Gain"=w190:T12, "Scan Mirror Position 1"=w204:T3, "Z Offset Position 1"=w203:T9, "Scan Mirror Position 2"=w202:T3, "Z Offset Position 2"=w201:T9, "Tuneable Lens 1"=w200:T13, "Tuneable Lens 2"=w199:T13, "Beam @ min Z"=w197:T3, "Beam @ max Z"=w198:T3, "Piezo Start (µm)"=w195:T4, "Piezo End (µm)"=w196:T4, "Number Z Slices"=w194:i16, "Filter Wheel Position"=w193:i32, "Apply ex/det correction"=w192:u16)  [unwired: 1 out]
        n338 = local write "MaxScanMirror"(w206) -> ()
        n339 = local write "Filter Wheel Position"(w193) -> ()
        n340 = local write "Apply ex/det correction"(w192) -> ()
        n341 = local write "PiezoEndMicrometres"(w196) -> ()
        n342 = local write "Number of Z Slices"(w194) -> ()
        n343 = local write "Lens 2"(w199) -> ()
        n344 = local write "@ max Z"(w198) -> ()
        n345 = local write "Lens 1"(w200) -> ()
        n346 = local write "Scan Mirror 1"(w204) -> ()
        n347 = local write "Scan Mirror 2"(w202) -> ()
        n348 = local write "Sample Rate (kHz)"(w208) -> ()
        n349 = local write "Laser"(w211) -> ()
        n350 = local write "Mirror Offset"(w191) -> ()
        n351 = local write "Z Mirror Gain"(w190) -> ()
        n352 = local write "Sweep Time (µS)"(w210) -> ()
        n353 = local write "@ min Z"(w197) -> ()
        n354 = local write "PiezoStartMicrometres"(w195) -> ()
        n355 = local write "MinScanMirror"(w205) -> ()
        n356 = local write "Z offset 2"(w201) -> ()
        n357 = local write "Z offset 1"(w203) -> ()
        n358 = local write "Sweep Interval (µS)"(w209) -> ()
        n359 = local write "Phase Shift (µS)"(w207) -> ()
      }
      event "loadMicroscopeSettings": Value Change {
        n360 = event-data() -> ()  [unwired: 1 in, 1 out]
        n361 = File Dialog(7:"Select Settings File " ("prompt")) -> (0:w222:errorcluster, 3:w220:path)  [unwired: 2 in, 6 out]
        n362 = Index Array(array=w218, index=0) -> (element=w219:T10)
        n363 = case shown="No Error" w222 {
          tunnel: w220 -> [w231 _]
          tunnel: w219 -> [w228 _]
          tunnel: [w224 w239] -> w217
          tunnel: w218 -> [_ w239]
          frame No Error {
            n364 = Open/Create/Replace Datalog(5:w228, 9:enum16{"read/write", "read-only", "write-only"}."read-only" ("access (0:read/write)"), 11:w231) -> (0:w238:errorcluster, 3:w229:refnum<k1>)  [unwired: 2 in, 2 out]
            n365 = Deny Access(4:w238, 6:T16."deny write-only" ("deny mode (0:deny read/write)"), 7:w229) -> (0:w237:errorcluster, 3:w236:refnum<k1>)
            n366 = Get Number of Records(4:w237, 7:w236) -> (0:w227:errorcluster, 2:w234:i64, 3:w235:refnum<k1>)
            n367 = Read Datalog(4:w227, 6:w234, 7:w235) -> (0:w226:errorcluster, 2:w224:T10[], 3:w233:refnum<k1>)
            n368 = Close File(refnum=w233, error in=w226) -> (error out=w232:errorcluster)  [unwired: 1 out]
            n369 = call <vilib>:"General Error Handler.vi"("error in (no error)"=w232) -> ()  [unwired: 4 in, 11 out]
          }
          frame Error {
          }
        }
      }
      event "saveMicroscopeSettings": Value Change {
        n370 = event-data() -> ()  [unwired: 1 in, 1 out]
        n371 = File Dialog(7:"Choose file name and location" ("prompt"), 9:"tunable lens settings.dat" ("default name")) -> (0:w244:errorcluster, 3:w243:path)  [unwired: 1 in, 6 out]
        n372 = Index Array(array=w240, index=0) -> (element=w241:T10)
        n373 = case shown="No Error" w244 {
          tunnel: w243 -> [w249 _]
          tunnel: w241 -> [w248 _]
          tunnel: w240 -> [w247 _]
          frame No Error {
            n374 = Open/Create/Replace Datalog(5:w248, 10:T17."replace or create" ("operation (0:open)"), 11:w249) -> (3:w252:refnum<k1>)  [unwired: 1 in, 4 out]
            n375 = for {
              tunnel: w247 -> [w258] mode=indexing
              tunnel: w252 -> [w257]
              tunnel: [w256] -> w251
              tunnel: [w255] -> w250
              n376 = Write Datalog(6:w258, 7:w257) -> (0:w255:errorcluster, 3:w256:refnum<k1>)  [unwired: 1 in]
            }
            n377 = Close File(refnum=w251, error in=w250) -> (error out=w254:errorcluster)  [unwired: 1 out]
            n378 = call <vilib>:"General Error Handler.vi"("error in (no error)"=w254) -> ()  [unwired: 1 in, 14 out]
          }
          frame Error {
          }
        }
      }
    }
    n379 = shared-variable "My Computer\\SharedVariables.lvlib\\COMport"("COM port") -> ()  [unwired: 1 in, 1 out]
    n380 = Unbundle By Name(w14) -> ("status"=w13:bool)
    n381 = local write "Microscope Settings"(w7) -> ()
    n382 = Or(x=w13, y=w16) -> (x .or. y?=w15:bool)
  }
  n383 = while {
    tunnel: w1 -> [w262]
    stop <- w259 stop-if-true
    # "This loop is a consumer loop."
    n384 = Dequeue Element(queue=w262) -> (element=w260:string, error out=w261:errorcluster)  [unwired: 2 in, 2 out]
    n385 = case shown="No Error" w261 {
      tunnel: w260 -> [w263 _]
      tunnel: [_ TRUE] -> w259
      frame No Error {
        n386 = case shown="\"manual\"" w263 {
          frame "SinglePlaneScan" {
            # "Process the data here."
            n387 = flat-sequence {
              frame #0 {
                n388 = shared-variable ".\\SharedVariables.lvlib\\StopSinglePlaneScan"(FALSE ("StopScan")) -> ()  [unwired: 1 in, 1 out]
              }
              frame #1 {
                n389 = while {
                  stop <- w265 stop-if-true
                  n390 = local read "Z offset 2"() -> (w270:T9)
                  n391 = local read "Mirror Offset"() -> (w269:dbl)
                  n392 = local read "Z Mirror Gain"() -> (w268:T6)
                  n393 = shared-variable ".\\SharedVariables.lvlib\\StopSinglePlaneScan"() -> (w265:bool)  [unwired: 1 in, 1 out]
                  n394 = local read "Piezo Position (µm)"() -> (w267:T8)
                  n395 = local read "@ max Z"() -> (w266:T3)
                  n396 = local read "Laser"() -> (w277:T7)
                  n397 = call "simple_scan_mathscript.vi"("Piezo"=w267, "Beam at max"=w266, "Laser"=w277, "Sweep Interval"="Sweep Interval (µS)", "Z mirror Gain"=w268, "Sample Rate"="Sample Rate (kHz)", "Z mirror offset"=w269, "Sweep Time"="Sweep Time (µS)", "Z offset 2"=w270, "Offset"="Offset", "Amplitude"="Amplitude", "Phase Shift"="Phase Shift (µS)") -> ()
                }
              }
            }
          }
          frame "MultiDScan" {
            n398 = flat-sequence {
              frame #0 {
                n399 = shared-variable ".\\SharedVariables.lvlib\\StopMultiDScan"(FALSE ("StopMultiDScan")) -> ()  [unwired: 1 in, 1 out]
              }
              frame #1 {
                n400 = call "multiD.vi"("Time Interval Between Repeats mS)"="Time Interval  Between Repeats (µS)", "Number of repetitions"="Number of Repetitions", "Array"="Microscope Settings") -> ()  [unwired: 9 in]
              }
              frame #2 {
                n401 = property on="StopMultiDScan" class="Bool"("DisabledEnum"=T15."Disabled and Grayed Out" ("Disabled")) -> ()  [unwired: 2 in, 2 out]
                n402 = property on="StartMultiDScan" class="Bool"("DisabledEnum"=T15."Enabled" ("Disabled")) -> ()  [unwired: 2 in, 2 out]
              }
            }
          }
          frame "manual" {
            n403 = call "mirrors_and_piezo_manual_scan.vi"("Stop Button"=FALSE) -> ()  [unwired: 1 in]
          }
          frame "other", Default {
          }
        }
      }
      frame Error {
        # "Return true in any case that should stop the loop."
      }
    }
  }
  n404 = Release Queue(queue=w1, error in (no error)=w4) -> ()  [unwired: 1 in, 3 out]
